vi "laneleftright5.vi"(11 "update":bool=TRUE) -> ()   [LabVIEW 2015]
uses:
  G_SEN.vi
  <vilib>/Analysis/1siggen.llb/Ramp Pattern by Delta.vi
  G_ALL.vi
  <vilib>/Analysis/polynomials.llb/nth Derivative of Polynomial (DBL).vi
  <vilib>/Analysis/polynomials.llb/Scalar Polynomial Evaluation (DBL).vi
  G_LCM.vi
  <vilib>/Analysis/NI_AALPro.lvlib
  <vilib>/Analysis/NI_AALBase.lvlib
panel:
  in  "y limit":dbl=0.01
  in  "d_safe front":dbl=0.5
  out "idxfront":i32=30
  out "h_rf":dbl[](array[numeric])=[-0.9500104358126387, -0.8152801995859489, -0.6832149509832309, -0.5579658214676491, -0.43634713174659895, -0.3636177945739105, -0.4219341557757026, -0.4254071654192556, -0.43418280012028193, -0.4285800458197435, -0.4285800458197435, -0.47492259541262927, -0.43011998989542144, -0.448140819410384, -0.42370272779821094, -0.4351070943600193, -0.3916639450286278, -0.31695052117940714, -0.29608961933059963, -0.29070058934802034, -0.19489158382745403, -0.13694705181123534, -0.0036604327923040465, 0.15093015758716827, 0.24134113354650677, 0.4371774287913892, 0.5886484511821607, 0.5886484511821607, 0.7188655986278671, 0.8431460626855709, 0.9539279580870911, 1.0615621391385646, 1.142586619661877, 1.1293783256575063, 1.1293783256600938, 1.1293783256589616, 1.129378308345949, 1.1293783256583803, 1.1293783256589178, 1.2328992187190753, 1.2383213544784377, 1.2299347078478895, 1.2485889663962422, 1.2492445630317817, 1.2507974714580428, 1.2535353037498, 1.2535353037498, 1.2548915682041502, 1.2388573722116965, 1.2551948137598792, 1.2561989169947274, 1.2545138672661875, 1.2372556012572844, 1.2374470995854208, 1.2497004386998842, 1.258883376955003, 1.238295612670253, 1.249261743063205, 1.2490590423907508, 1.2394351036162379, 1.249147146451496, 1.2523281510667994, 1.2568185177320512, 1.2637485927398984, 1.2729524270473782, 1.2872258426538232, 1.3082533285080937, 1.3356267808199382, 1.3717983894543175, 1.4090203881905266, 1.496939359193244, 1.5483512846148995, 1.5906635102611244, 1.5906635102611244, 1.5906635102611244, 1.5906635102611244, 1.5906635102611244, 1.5906635102611244, 1.5906635102611244, 1.5906635102611244, 1.5906635102611244]
  out "h_lf":dbl[](array[numeric])=[-1.07768170874119, -0.9500104358126387, -0.8152801995859489, -0.6832149509832309, -0.5579658214676491, -0.43634713174659895, -0.3636177945739105, -0.38220962901672345, -0.4254071654192556, -0.43418280012028193, -0.4285800458197435, -0.47492259541262927, -0.43011998989542144, -0.448140819410384, -0.42370272779821094, -0.4351070943600193, -0.3916639450286278, -0.3566256576667743, -0.31695052117940714, -0.29608961933059963, -0.29070058934802034, -0.19489158382745403, -0.13694705181123534, -0.0036604327923040465, 0.15093015758716827, 0.15093015758716827, 0.24134113354650677, 0.4371774287913892, 0.5886484511821607, 0.7188655986278671, 0.8431460626855709, 0.9539279580870911, 1.0615621391385646, 1.142586619661877, 1.1504547666405178, 1.1293783256600938, 1.1293783256589616, 1.1293783256583803, 1.1293783256589178, 1.2328992187190753, 1.2383213544784377, 1.2299347078478895, 1.2299347078478895, 1.2485889663962422, 1.2492445630317817, 1.2507974714580428, 1.2535353037498, 1.2548915682041502, 1.2388573722116965, 1.2551948137598792, 1.2561989169947274, 1.2545138672661875, 1.2372556012572844, 1.2374470995854208, 1.2497004386998842, 1.258883376955003, 1.238295612670253, 1.249261743063205, 1.2490590423907508, 1.2394351036162379, 1.249147146451496, 1.2523281510667994, 1.2568185177320512, 1.2637485927398984, 1.2729524270473782, 1.2872258426538232, 1.3082533285080937, 1.3356267808199382, 1.3717983894543175, 1.4090203881905266, 1.4509264137298254, 1.496939359193244, 1.5483512846148995, 1.5906635102611244, 1.5906635102611244, 1.5906635102611244, 1.5906635102611244, 1.5906635102611244, 1.5906635102611244, 1.5906635102611244, 1.5906635102611244]
  out "size limit":i32=75
  out "sorted array":dbl[](array[numeric])=[3.1256999216175574, 3.1400636936215167, 3.178049716414141, 3.178049716414141, 3.1953090617340916, 3.2015621187164243, 3.2015621187164247, 3.2015621187164247, 3.22490309931942, 3.228002478313795, 3.2280024783137953, 3.2310988842807027, 3.23882694814033, 3.2557641192199416, 3.2557641192199416, 3.2557641192199416, 3.2572994949804666, 3.264965543462902, 3.269556544854363, 3.2756678708318403, 3.2756678708318403, 3.2893768406797053, 3.2893768406797057, 3.298484500494129, 3.298484500494129, 3.298484500494129, 3.301514803843836, 3.306055050963308, 3.3105890714493698, 3.3120990323358392, 3.3136083051561784, 3.3241540277189325, 3.3241540277189325, 3.3241540277189325, 3.3241540277189325, 3.3241540277189325, 3.324154027718933, 3.3376638536557275, 3.3526109228480423, 3.3526109228480423, 3.3526109228480423, 3.3526109228480423, 3.3541019662496847, 3.3541019662496847, 3.361547262794322, 3.361547262794323, 3.383784863137726, 3.3837848631377265, 3.3837848631377265, 3.4, 3.4000000000000004, 3.4000000000000004, 3.400000000000001, 3.4014702703389896, 3.40147027033899, 3.4014702703389905, 3.4132096331752027, 3.417601498127013, 3.417601498127013, 3.417601498127013, 3.4438350715445134, 3.448187929913334, 3.448187929913334, 3.4481879299133342, 3.453983207834109, 3.4669871646719437, 3.4669871646719437, 3.4785054261852175, 3.4785054261852175, 3.4885527085024823, 3.4928498393145966, 3.4985711369071804, 3.511409973215888, 3.5227829907617076, 3.534119409414459, 3.535533905932738, 3.5510561809129415, 3.5777087639996643, 3.580502757993632, 3.5846896657869842, 3.6055512754639896, 3.6235341863986887, 3.635931792539569, 3.6400549446402595, 3.6619666847201118, 3.6878177829171555, 3.7013511046643504, 3.720215047547655, 3.753664875824692, 3.764306044943743, 3.8288379438153295]
  out "element":dbl=2.140625
  out "size(s) 4":i32=91
  out "size(s) 3":i32=52
  in  "x limit":dbl=0.01
  in  "x_gain":dbl=0.5
  out "xr":dbl[](array[numeric])=[2.3000000000000003, 2.3000000000000003, 2.3000000000000003, 2.3000000000000003, 2.3000000000000003, 2.3000000000000003, 2.2, 2.2, 2.2, 2.2, 2.2, 2.2, 2.2, 2.2, 2.2, 2.1, 2.1, 2.1, 2.1, 2.1, 2.1, 2.0, 2.0, 1.9000000000000001, 1.9000000000000001, 1.8, 1.8, 1.8, 1.8, 1.8, 1.7000000000000002, 1.7000000000000002, 1.7000000000000002, 1.7000000000000002, 1.7000000000000002, 1.7000000000000002, 1.7000000000000002, 1.7000000000000002, 1.7000000000000002, 1.7000000000000002, 1.7000000000000002, 1.7000000000000002, 1.7000000000000002, 1.7000000000000002, 1.6, 1.6, 1.6, 1.6, 1.6, 1.6]
  out "yr":dbl[](array[numeric])=[-2.0, -2.1, -2.2, -2.3000000000000003, -2.4000000000000004, -2.5, 1.7000000000000002, 1.6, 1.5, -1.7000000000000002, -1.8, -1.9000000000000001, -2.0, -2.1, -2.2, 1.5, -1.5, -1.6, -1.7000000000000002, -1.8, -1.9000000000000001, -1.5, -1.6, -1.1, -1.2000000000000002, -0.6000000000000001, -0.7000000000000001, -0.8, -1.1, -1.2000000000000002, 0.8, 0.7000000000000001, 0.6000000000000001, 0.5, 0.4, 0.30000000000000004, -0.1, -0.2, -0.30000000000000004, -0.4, -0.5, -0.6000000000000001, -0.7000000000000001, -0.8, 0.4, 0.30000000000000004, 0.2, -0.1, -0.2, -0.30000000000000004]
  out "yl":dbl[](array[numeric])=[-4.800000000000001, -4.9, -5.0, -4.4, -4.5, -4.6000000000000005, -4.7, -4.800000000000001, -4.9, -5.0, -4.1000000000000005, -4.2, -4.3, -4.4, -4.5, -4.6000000000000005, -4.7, -3.7, -3.8000000000000003, -3.9000000000000004, -4.0, -4.1000000000000005, -4.2, -4.3, -4.4, -3.5, -3.6, -3.7, -3.8000000000000003, -3.9000000000000004, -4.0, -4.1000000000000005, -3.0, -3.1, -3.2, -3.3000000000000003, -3.4000000000000004, -3.5, -3.6, -3.7, -2.7, -2.8000000000000003, -2.9000000000000004, -3.0, -3.1, -3.2, -3.3000000000000003, -2.3000000000000003, -2.4000000000000004, -2.5, -2.6, -2.7, -2.8000000000000003, -1.9000000000000001, -2.0, -2.1, -2.2, -2.3000000000000003, -2.4000000000000004, -2.5, -2.6, -1.2000000000000002, -1.3, -1.5, -1.6, -1.7000000000000002, -1.8, -1.9000000000000001, -2.0, -2.1, -2.2, -1.1, -1.2000000000000002, -1.4000000000000001, -1.5, -1.6, -1.7000000000000002, -0.8, -0.9, -1.1, -0.4, -0.5, -0.6000000000000001, -0.7000000000000001, -0.8, -0.9, -0.2, -0.30000000000000004, -0.4]
  out "xl":dbl[](array[numeric])=[-0.5, -0.5, -0.5, -0.6000000000000001, -0.6000000000000001, -0.6000000000000001, -0.6000000000000001, -0.6000000000000001, -0.6000000000000001, -0.6000000000000001, -0.7000000000000001, -0.7000000000000001, -0.7000000000000001, -0.7000000000000001, -0.7000000000000001, -0.7000000000000001, -0.7000000000000001, -0.8, -0.8, -0.8, -0.8, -0.8, -0.8, -0.8, -0.8, -0.9, -0.9, -0.9, -0.9, -0.9, -0.9, -0.9, -1.0, -1.0, -1.0, -1.0, -1.0, -1.0, -1.0, -1.0, -1.1, -1.1, -1.1, -1.1, -1.1, -1.1, -1.1, -1.2000000000000002, -1.2000000000000002, -1.2000000000000002, -1.2000000000000002, -1.2000000000000002, -1.2000000000000002, -1.3, -1.3, -1.3, -1.3, -1.3, -1.3, -1.3, -1.3, -1.4000000000000001, -1.4000000000000001, -1.4000000000000001, -1.4000000000000001, -1.4000000000000001, -1.4000000000000001, -1.4000000000000001, -1.4000000000000001, -1.4000000000000001, -1.4000000000000001, -1.5, -1.5, -1.5, -1.5, -1.5, -1.5, -1.6, -1.6, -1.6, -1.7000000000000002, -1.7000000000000002, -1.7000000000000002, -1.7000000000000002, -1.7000000000000002, -1.7000000000000002, -1.8, -1.8, -1.8]
  out "lf_shift":dbl
  out "lr_shift":dbl
  out "rf_shift":dbl
  out "rr_shift":dbl
  in  "y_gain":dbl=0.5
  out "y_shift":dbl format="%#_13g"
  out "x_shift":dbl format="%#_13g"
  in  "d_safe":dbl=0.25
  out "R0":dbl=3.023957560629749
  out "y_ramp":dbl[](array[numeric])=[-1.0, -0.75, -0.5, -0.25, 0.0, 0.25, 0.5, 0.75, 1.0, 1.25, 1.5, 1.75, 2.0, 2.25, 2.5, 2.75, 3.0, 3.25, 3.5, 3.75, 4.0, 4.25, 4.5, 4.75, 5.0, 5.25, 5.5, 5.75, 6.0]
  out "y_car":dbl[](array[numeric])=[0.0, 3.2, 3.2, 0.0, 0.0]
  out "x_car":dbl[](array[numeric])=[0.8, 0.8, -0.8, -0.8, 0.8]
  out "x_rf":dbl[](array[numeric])=[4.538572328164872, 4.118234620393652, 3.7108458254827896, 3.3870811007829085, 3.120851291928107, 2.916943626318998, 2.7777005691770915, 2.725587769939431, 2.739475625042867, 2.8048150174077966, 2.925745330134693, 2.950997308985372, 2.7112467821790673, 2.394172481092407, 2.174401406783209, 1.9364338560710306, 1.7440716120528545, 1.385310657465475, 1.3006647210601057, 1.0310989075140025, 0.886404618470291, 0.643840438515097, 0.5740896815265153, 0.49712084094748343, 0.45274653237776485, 0.36494746145204304, 0.2359651958610256, 0.40853962746891925, 0.501296155076003, 0.865183184427989, 1.3470915265169374, 1.6921924502018477, 2.350947359675299, 2.926007032436896, 3.472919068553876, 4.01553923764964, 4.540771553603303, 5.060339948090165, 5.558610823136398, 6.019770740590945, 6.466417913813986, 6.886028933795981, 7.305639953774969, 7.725250962609034, 8.144861995684934, 8.564473015664918, 9.033292240733939, 9.507748305528745, 9.982559003445736, 10.465812099477526, 10.944605083330368, 11.422232043345485, 11.918421793799222, 12.414200190202452, 12.899637481676528, 13.37678754684273, 13.874783465668319, 14.370744561954087, 14.868407110563963, 15.347734850377055, 15.829260577613933, 16.33800747711995, 16.840800167460728, 17.330629454236842, 17.83149600020578, 18.307170795470793, 18.793936003289474, 19.282694540287146, 19.78369621145204, 20.267635515491328, 20.756809613631752, 21.25179974157784, 21.74713849772317, 22.236508427679524, 22.722656802659756, 23.209593805045373, 23.694584083823898, 24.18159320732069, 24.656670896067542, 25.139986749461006, 25.646977091436657]
  out "y_rf":dbl[](array[numeric])=[-11.133801995366914, -10.775342355485478, -10.460977313011862, -10.008167510844103, -9.519733334433447, -9.006779742303703, -8.476797423718132, -7.920018039425989, -7.363784000331509, -6.820753362891501, -6.29243806249853, -5.801400680342903, -5.33902916891923, -4.892670984988988, -4.430237539433438, -3.9731282342132452, -3.5156906037336335, -3.0892706515763058, -2.6129748065047353, -2.163986278307514, -1.6831045571753158, -1.2341811741681994, -0.7562032880817622, -0.27746062806621064, 0.20341311916780747, 0.6846965145469994, 1.1665722299824774, 1.6449603307709209, 2.125056894695668, 2.5475589084455996, 2.8962835690170365, 3.265562716322244, 3.4006089292605273, 3.512279221773241, 3.5953374904708157, 3.622437769324544, 3.623063809872327, 3.5757747817018526, 3.56036016701454, 3.743209849888086, 4.016917878895559, 4.215189945468877, 4.413462012052612, 4.61173413464184, 4.810006155024352, 5.008278221603526, 4.868806594115014, 5.017139252390996, 5.209509379461617, 5.317736171223016, 5.47536534066575, 5.629232093137066, 5.784437062614739, 5.942659837296325, 6.155411787532055, 6.264698912841051, 6.42392237988264, 6.590981837822474, 6.812082411109792, 6.977514156959353, 7.102822406709091, 7.24110252096422, 7.472616124159055, 7.604691291930131, 7.772210321235591, 7.963262450759516, 8.097906275068672, 8.250045548981548, 8.40009947677207, 8.53394808955574, 8.658191795172698, 8.762449905848245, 8.8369058516278, 8.878040735642243, 8.876062057147013, 8.853346181102042, 8.797375639621363, 8.708634139574771, 8.579950576586779, 8.456123819728742, 8.446050024161806]
  out "y_rr":dbl[](array[numeric])=[-10.70948639810373, -10.768851501394227, -10.773698390308322, -10.742191022481514, -10.657439960127398, -10.52156928101113, -10.338156146215423, -10.114144305421542, -9.845534928412233, -9.535421794598271, -9.192602940142088, -8.792172667355606, -8.308126041009189, -7.812026379085751, -7.345024018399936, -6.876213405347107, -6.426272269508127, -5.935120632545394, -5.521505119616947, -5.047999798768626, -4.600137704349835, -4.136020874717464, -3.7138838228732727, -3.2761172269068966, -2.837195735363109, -2.3760547770738345, -1.8991663469164366, -1.4944594171009975, -1.0449827814742285, -0.6524196535491742, -0.2673377084370725, 0.15830412292045987, 0.5015679626686349, 0.8508652409058738, 1.187167083685631, 1.4940639050112943, 1.771916455237049, 2.0157467968022704, 2.231583141944811, 2.437378476871852, 2.6498075579368594, 2.848079624517664, 3.0463516910981228, 3.2446237635961372, 3.442895834068181, 3.6411679006489104, 3.8079942899104933, 3.972712173496366, 4.139751736152054, 4.304420660079245, 4.464039995334728, 4.6226225761415085, 4.786147622632705, 4.948494763708864, 5.1126061835115255, 5.271456251848721, 5.43373465243814, 5.595668001049872, 5.764432278430686, 5.930443066452188, 6.09288119931919, 6.259087021699353, 6.428111182822922, 6.59341810511168, 6.760321754935594, 6.922204842602915, 7.086285179001638, 7.248086732121628, 7.411797351666064, 7.566761628321898, 7.719120690821865, 7.867136904452785, 8.006386664257533, 8.132415557859344, 8.243463199248932, 8.337918310717816, 8.414709864120713, 8.472506653347954, 8.508132472051695, 8.519694624675884, 8.509620829108949]
  out "x_rr":dbl[](array[numeric])=[7.710315740535928, 7.318228037388939, 6.895528781102477, 6.501757566222534, 6.111774833888363, 5.735704462825447, 5.380649609435707, 5.054924570161421, 4.7596024356590885, 4.499092239675365, 4.278166744665951, 4.089102278529083, 3.904755795193055, 3.7046548666886947, 3.495014818056198, 3.282575189342792, 3.0739266292849514, 2.848573410978404, 2.6350002926864415, 2.4176291141079678, 2.2020480421551136, 1.9926645012883535, 1.7956157164989206, 1.6142862728460952, 1.4500919057305408, 1.2986505892402076, 1.1531603649029383, 1.028252179118328, 0.9381582059669654, 0.8768965432058912, 0.8659466285499812, 0.9273761103327463, 0.9961184132684305, 1.1492471661511572, 1.365618593566012, 1.6259734415878775, 1.9305505914189107, 2.2663620157631854, 2.647536860206764, 3.0983319811358476, 3.573148246062948, 3.9927592660414053, 4.412370286021941, 4.8319813185248055, 5.251592327932702, 5.67120334791195, 6.014239863704302, 6.482988467645475, 6.9666646776145456, 7.430488117614067, 7.908617427576298, 8.384677553250869, 8.878122763437181, 9.372550012016466, 9.874318246914124, 10.334836032372968, 10.831836166680331, 11.329470097797818, 11.84476209179978, 12.323889263806183, 12.792812198731816, 13.29241302624446, 13.816067216021146, 14.294624424329601, 14.795696018423165, 15.281249604081424, 15.758046881797691, 16.24360281259667, 16.740135975558726, 17.21729941118971, 17.697701008012572, 18.179599450331803, 18.656792581905684, 19.124588908434816, 19.585808275078925, 20.051376885574644, 20.517546642391945, 20.99031700331575, 21.45747691009842, 21.940618256655217, 22.447608598630868]
  out "x_lr":dbl[](array[numeric])=[7.9224735391675205, 7.321473464434564, 6.739168242454245, 6.134745810403829, 5.542921521041388, 4.978309693471735, 4.449970248187061, 3.9578614371636447, 3.5187269716187273, 3.14175802382198, 2.8280843058441714, 2.5937162850227318, 2.4202073591480753, 2.244977169640313, 2.0376215785729492, 1.8310326037758613, 1.6186357963977047, 1.42564842049386, 1.1807351361303358, 0.9756223538774118, 0.7435314685678545, 0.5417446510137208, 0.31677544910316535, 0.1149579734257522, -0.0702125215349173, -0.23172505657020925, -0.37970892354651875, -0.5414576948176312, -0.6468616321179829, -0.7230927377914959, -0.7158640101770734, -0.6262531863681458, -0.45340207002751576, -0.18145982428252616, 0.16153339017341928, 0.5617865094312524, 1.0049769141012719, 1.4863480233133943, 1.9831483476718994, 2.4454162946277305, 2.889593085583598, 3.309204105565798, 3.7288151255446973, 4.148426133001953, 4.568037167454616, 4.987648187434642, 5.483833711602041, 5.960774928198159, 6.431785855959763, 6.923830362042183, 7.402954754910787, 7.88137279475309, 8.378978043446166, 8.875467475222736, 9.352915444903859, 9.838214701876803, 10.336742302958081, 10.831813179411517, 11.320937025460228, 11.8003537185526, 12.287841595036866, 12.801405276612027, 13.293814745353078, 13.788987830920377, 14.289751735273168, 14.760720800003124, 15.252236333764175, 15.74262340416671, 16.245984913005724, 16.733706180572792, 17.228165455837157, 17.73194294963407, 18.24153298822055, 18.751776319543367, 19.26950884612988, 19.79366295038253, 20.326213754641618, 20.87225326020234, 21.42156785783088, 21.97240365912879, 22.479394001104442]
  out "y_lr":dbl[](array[numeric])=[-12.295358104289258, -12.368848209891869, -12.366039868118165, -12.299529255201328, -12.152901731107526, -11.930949699264355, -11.63963066634473, -11.278812705532536, -10.855598333720343, -10.382560405732054, -9.868813647407716, -9.361225152127462, -8.904880547516182, -8.467267571883895, -8.005330724036432, -7.549284071982989, -7.0911997781241745, -6.666752009301859, -6.188672905430115, -5.741264902065608, -5.257959416192246, -4.810432906104093, -4.324646840359476, -3.834699942856202, -3.3358684220394967, -2.8429063409679163, -2.357763931437393, -1.8043156929257018, -1.2634138069197096, -0.6582763329381254, -0.026765259453594398, 0.5407122928550108, 1.178982435872069, 1.7392451740487433, 2.240817321179563, 2.6888468030421757, 3.0770269363292453, 3.4127357629657604, 3.6871201234096276, 3.898097856599401, 4.096442391812379, 4.294714458394951, 4.492986524974636, 4.691258585638252, 4.889530667944297, 5.087802734525394, 5.317520478425312, 5.485092092438001, 5.64769889906765, 5.822082651010975, 5.982033823211763, 6.141399821188817, 6.306297137813725, 6.469319852801857, 6.625265800892727, 6.792432009083602, 6.955208301932135, 7.116305233128007, 7.276254787812777, 7.442365859737624, 7.611105388760248, 7.781884247137096, 7.940477658542712, 8.1114206200653, 8.278221745826903, 8.4351654382976, 8.604229739747527, 8.767632595966866, 8.93357746961272, 9.091929680472706, 9.248674993631454, 9.403237050075806, 9.551559622166277, 9.688375317481698, 9.811887463039348, 9.917026770453182, 10.003228584836691, 10.068144755350426, 10.107729465036254, 10.119378871078778, 10.109305075511843]
  out "af":dbl=3.2
  out "y_lf":dbl[](array[numeric])=[-12.719673701552441, -12.375339063983121, -12.053318790821704, -11.565505743563916, -11.015195105413575, -10.416160160556927, -9.77827194384744, -9.084686439536984, -8.37384740563962, -7.667891974025285, -6.968648769764158, -6.370453165114759, -5.935783675426223, -5.547912177787132, -5.090544245069932, -4.646198900849126, -4.180618112349682, -3.82090202833277, -3.280142592317903, -2.8572513816044967, -2.340926269017727, -1.9085932055548271, -1.3669663055679653, -0.8360433440155162, -0.2952595675085803, 0.21784495065291676, 0.7079746454615212, 1.3351040549462165, 1.906625869250187, 2.5417022290566487, 3.1368560180005147, 3.6479708862567946, 4.078023402463962, 4.40065915491611, 4.648987727964748, 4.817220667355426, 4.928174290964523, 4.9727637478653435, 5.0158971484793575, 5.2039292296156345, 5.463552712771079, 5.661824779346166, 5.860096845929126, 6.058368956683955, 6.256640988900468, 6.45491305548001, 6.378332782629832, 6.529519171332631, 6.717456542377213, 6.835398162154745, 6.993359168542785, 7.148009338184375, 7.304586577795758, 7.4634849263893175, 7.668071404913257, 7.785674670075932, 7.945396029376635, 8.111619069900609, 8.323904920491882, 8.489436950244789, 8.62104659615015, 8.763899746401965, 8.984982599878846, 9.122693806883749, 9.290110312126899, 9.476223046454201, 9.615850835814562, 9.769591412826784, 9.921879594718726, 10.059116141706546, 10.187746097982288, 10.298550051471265, 10.382078809536544, 10.434000495264597, 10.44448632093743, 10.432454640837406, 10.385894360337339, 10.304272241577243, 10.179547569571339, 10.055808066131636, 10.0457342705647]
  out "x_lf":dbl[](array[numeric])=[4.750730126796465, 4.121480047439278, 3.5544852868345593, 3.0200693449642024, 2.5519979790811314, 2.159548856965284, 1.847021207928445, 1.628524636941655, 1.4986001610025053, 1.4474808015544118, 1.4756628913129135, 1.455611315479021, 1.226698346134088, 0.9344947840440256, 0.7170081672999595, 0.48489127050409975, 0.28878077916560807, -0.037614333019069246, -0.15360043549600033, -0.4109078527165533, -0.5721119551169682, -0.8070794117595357, -0.90475058586924, -1.0022074584728595, -1.0675578948876934, -1.1654281843583738, -1.2969040925884314, -1.16117024646704, -1.0837236830089454, -0.734806096569398, -0.23471911221011726, 0.13856315350095594, 0.9014268763793528, 1.5953000420032126, 2.2688338651612834, 2.951352305493015, 3.615197876285664, 4.280325955640375, 4.894222310601533, 5.366855054082828, 5.782862753334636, 6.202473773320374, 6.6220847932977245, 7.041695777086183, 7.461306835206849, 7.88091785518761, 8.502886088631676, 8.98553476608143, 9.447680181790954, 9.95915434390564, 10.438942410664858, 10.918927284847708, 11.419277073808205, 11.917117653408722, 12.378234679666264, 12.880166216346565, 13.379689601946069, 13.873087643567787, 14.34458204422441, 14.824199305123472, 15.324289973918983, 15.846999727487516, 16.31854769679266, 16.824992860827617, 17.325551717055784, 17.786641991392493, 18.288125455255955, 18.781715131857183, 19.289545148899034, 19.784042284874406, 20.287274061456333, 20.804143240880112, 21.33187890403804, 21.863695838788075, 22.406357373710716, 22.951879869853258, 23.50325119607357, 24.063529464207285, 24.6207618438, 25.171772151934576, 25.678762493910227]
  out "h_path":dbl[](array[numeric])=[-1.7037866247771944, -1.5728247200893424, -1.4729147677282362, -1.3393532640375114, -1.2073117198254844, -1.07768170874119, -0.9500104358126387, -0.8152801995859489, -0.6832149509832309, -0.5579658214676491, -0.43634713174659895, -0.3636177945739105, -0.38220962901672345, -0.4219341557757026, -0.4254071654192556, -0.43418280012028193, -0.4285800458197435, -0.47492259541262927, -0.43011998989542144, -0.448140819410384, -0.42370272779821094, -0.4351070943600193, -0.3916639450286278, -0.3566256576667743, -0.31695052117940714, -0.29608961933059963, -0.29070058934802034, -0.19489158382745403, -0.13694705181123534, -0.0036604327923040465, 0.15093015758716827, 0.24134113354650677, 0.4371774287913892, 0.5886484511821607, 0.7188655986278671, 0.8431460626855709, 0.9539279580870911, 1.0615621391385646, 1.142586619661877, 1.1504547666405178, 1.1293783256575063, 1.1293783256600938, 1.1293783256589616, 1.129378308345949, 1.1293783256583803, 1.1293783256589178, 1.2328992187190753, 1.2383213544784377, 1.2299347078478895, 1.2485889663962422, 1.2492445630317817, 1.2507974714580428, 1.2535353037498, 1.2548915682041502, 1.2388573722116965, 1.2551948137598792, 1.2561989169947274, 1.2545138672661875, 1.2372556012572844, 1.2374470995854208, 1.2497004386998842, 1.258883376955003, 1.238295612670253, 1.249261743063205, 1.2490590423907508, 1.2394351036162379, 1.249147146451496, 1.2523281510667994, 1.2568185177320512, 1.2637485927398984, 1.2729524270473782, 1.2872258426538232, 1.3082533285080937, 1.3356267808199382, 1.3717983894543175, 1.4090203881905266, 1.4509264137298254, 1.496939359193244, 1.5483512846148995, 1.5906635102611244, 1.5906635102611244]
  out "x_path":dbl[](array[numeric])=[7.816394639851724, 7.319850750911751, 6.817348511778361, 6.318251688313182, 5.827348177464875, 5.357007078148591, 4.915309928811384, 4.506393003662533, 4.139164703638908, 3.8204251317486726, 3.553125525255061, 3.3414092817759076, 3.162481577170565, 2.974816018164504, 2.7663181983145737, 2.5568038965593267, 2.346281212841328, 2.137110915736132, 1.9078677144083886, 1.6966257339926898, 1.4727897553614842, 1.267204576151037, 1.056195582801043, 0.8646221231359237, 0.6899396920978118, 0.5334627663349991, 0.38672572067820976, 0.24339724215034841, 0.1456482869244913, 0.07690190270719764, 0.07504130918645387, 0.15056146198230025, 0.2713581716204574, 0.48389367093431557, 0.7635759918697156, 1.093879975509565, 1.4677637527600913, 1.8763550195382899, 2.3153426039393317, 2.771874137881789, 3.231370665823273, 3.6509816858036017, 4.070592705783319, 4.490203725763379, 4.909814747693659, 5.329425767673296, 5.749036787653171, 6.221881697921817, 6.699225266787154, 7.177159239828125, 7.6557860912435425, 8.133025174001979, 8.628550403441674, 9.124008743619601, 9.613616845908991, 10.086525367124885, 10.584289234819206, 11.080641638604668, 11.582849558630004, 12.062121491179392, 12.540326896884341, 13.046909151428244, 13.554940980687112, 14.041806127624989, 14.542723876848166, 15.020985202042274, 15.505141607780933, 15.99311310838169, 16.493060444282225, 16.97550279588125, 17.462933231924865, 17.955771199982937, 18.449162785063116, 18.938182613989092, 19.427658560604403, 19.922519917978587, 20.42188019851678, 20.931285131759044, 21.43952238396465, 21.956510957892004, 22.463501299867655]
  out "y_path":dbl[](array[numeric])=[-11.502422251196494, -11.568849855643048, -11.569869129213243, -11.520860138841421, -11.405170845617462, -11.226259490137743, -10.988893406280077, -10.696478505477039, -10.350566631066288, -9.958991100165163, -9.530708293774902, -9.076698909741534, -8.606503294262685, -8.139646975484823, -7.675177371218184, -7.212748738665048, -6.758736023816151, -6.300936320923626, -5.855089012523531, -5.394632350417117, -4.92904856027104, -4.473226890410778, -4.019265331616374, -3.5554085848815493, -3.086532078701303, -2.6094805590208754, -2.1284651391769147, -1.6493875550133497, -1.154198294196969, -0.6553479932436498, -0.14705148394533343, 0.3495082078877353, 0.840275199270352, 1.2950552074773085, 1.7139922024325969, 2.091455354026735, 2.424471695783147, 2.7142412798840154, 2.9593516326772193, 3.1677381667356266, 3.373124974874619, 3.571397041456308, 3.76966910803638, 3.9679411746171946, 4.166213251006239, 4.364485317587152, 4.562757384167902, 4.728902132967184, 4.893725317609852, 5.06325165554511, 5.223036909273246, 5.382011198665163, 5.546222380223215, 5.708907308255361, 5.868935992202126, 6.031944130466162, 6.194471477185138, 6.35598661708894, 6.520343533121731, 6.686404463094906, 6.851993294039719, 7.0204856344182245, 7.184294420682817, 7.35241936258849, 7.5192717503812485, 7.678685140450257, 7.845257459374583, 8.007859664044247, 8.172687410639393, 8.329345654397303, 8.483897842226659, 8.635186977264295, 8.778973143211905, 8.910395437670521, 9.02767533114414, 9.127472540585499, 9.208969224478702, 9.27032570434919, 9.307930968543975, 9.319536747877331, 9.309462952310396]
  out "gap":dbl=0.8
  out "theta":dbl[](array[numeric])=[-3.141592653589793, -3.1315926535897933, -3.121592653589793, -3.1115926535897933, -3.101592653589793, -3.0915926535897933, -3.081592653589793, -3.0715926535897933, -3.061592653589793, -3.0515926535897933, -3.041592653589793, -3.0315926535897932, -3.021592653589793, -3.0115926535897932, -3.001592653589793, -2.991592653589793, -2.981592653589793, -2.971592653589793, -2.961592653589793, -2.951592653589793, -2.941592653589793, -2.931592653589793, -2.921592653589793, -2.911592653589793, -2.901592653589793, -2.891592653589793, -2.8815926535897933, -2.871592653589793, -2.861592653589793, -2.851592653589793, -2.8415926535897933, -2.831592653589793, -2.8215926535897933, -2.811592653589793, -2.8015926535897933, -2.791592653589793, -2.7815926535897932, -2.771592653589793, -2.7615926535897932, -2.751592653589793, -2.741592653589793, -2.731592653589793, -2.721592653589793, -2.711592653589793, -2.701592653589793, -2.691592653589793, -2.681592653589793, -2.671592653589793, -2.661592653589793, -2.651592653589793, -2.641592653589793, -2.6315926535897933, -2.621592653589793, -2.611592653589793, -2.601592653589793, -2.5915926535897933, -2.581592653589793, -2.571592653589793, -2.561592653589793, -2.5515926535897933, -2.541592653589793, -2.5315926535897932, -2.521592653589793, -2.5115926535897932, -2.501592653589793, -2.491592653589793, -2.481592653589793, -2.471592653589793, -2.461592653589793, -2.451592653589793, -2.441592653589793, -2.431592653589793, -2.4215926535897934, -2.411592653589793, -2.401592653589793, -2.391592653589793, -2.3815926535897933, -2.371592653589793, -2.361592653589793, -2.351592653589793, -2.3415926535897933, -2.331592653589793, -2.321592653589793, -2.311592653589793, -2.3015926535897933, -2.291592653589793, -2.2815926535897932, -2.271592653589793, -2.2615926535897932, -2.251592653589793, -2.241592653589793, -2.231592653589793, -2.221592653589793, -2.211592653589793, -2.201592653589793, -2.191592653589793, -2.181592653589793, -2.1715926535897934, -2.161592653589793, -2.151592653589793, -2.141592653589793, -2.1315926535897933, -2.121592653589793, -2.111592653589793, -2.101592653589793, -2.0915926535897933, -2.081592653589793, -2.071592653589793, -2.061592653589793, -2.0515926535897933, -2.041592653589793, -2.031592653589793, -2.021592653589793, -2.0115926535897932, -2.001592653589793, -1.991592653589793, -1.9815926535897932, -1.9715926535897932, -1.9615926535897932, -1.9515926535897932, -1.9415926535897932, -1.9315926535897932, -1.9215926535897931, -1.9115926535897931, -1.9015926535897931, -1.8915926535897931, -1.881592653589793, -1.871592653589793, -1.861592653589793, -1.851592653589793, -1.841592653589793, -1.831592653589793, -1.821592653589793, -1.811592653589793, -1.801592653589793, -1.791592653589793, -1.781592653589793, -1.771592653589793, -1.761592653589793, -1.751592653589793, -1.741592653589793, -1.7315926535897932, -1.7215926535897932, -1.7115926535897932, -1.7015926535897932, -1.6915926535897932, -1.6815926535897932, -1.6715926535897931, -1.6615926535897931, -1.6515926535897931, -1.6415926535897931, -1.631592653589793, -1.621592653589793, -1.611592653589793, -1.601592653589793, -1.591592653589793, -1.581592653589793, -1.571592653589793, -1.561592653589793, -1.551592653589793, -1.541592653589793, -1.531592653589793, -1.521592653589793, -1.511592653589793, -1.501592653589793, -1.491592653589793, -1.481592653589793, -1.4715926535897932, -1.4615926535897932, -1.4515926535897932, -1.4415926535897932, -1.4315926535897932, -1.4215926535897931, -1.4115926535897931, -1.4015926535897931, -1.3915926535897931, -1.381592653589793, -1.371592653589793, -1.361592653589793, -1.351592653589793, -1.341592653589793, -1.331592653589793, -1.321592653589793, -1.311592653589793, -1.301592653589793, -1.291592653589793, -1.281592653589793, -1.271592653589793, -1.261592653589793, -1.251592653589793, -1.241592653589793, -1.231592653589793, -1.2215926535897932, -1.2115926535897932, -1.2015926535897932, -1.1915926535897932, -1.1815926535897932, -1.1715926535897931, -1.1615926535897931, -1.1515926535897931, -1.1415926535897931, -1.1315926535897929, -1.121592653589793, -1.1115926535897929, -1.101592653589793, -1.0915926535897933, -1.081592653589793, -1.0715926535897933, -1.061592653589793, -1.0515926535897933, -1.041592653589793, -1.0315926535897932, -1.021592653589793, -1.0115926535897932, -1.001592653589793, -0.9915926535897932, -0.981592653589793, -0.9715926535897932, -0.961592653589793, -0.9515926535897932, -0.9415926535897929, -0.9315926535897932, -0.9215926535897929, -0.9115926535897931, -0.9015926535897929, -0.8915926535897931, -0.8815926535897929, -0.8715926535897931, -0.8615926535897929, -0.8515926535897931, -0.8415926535897928, -0.8315926535897931, -0.8215926535897933, -0.811592653589793, -0.8015926535897933, -0.791592653589793, -0.7815926535897932, -0.771592653589793, -0.7615926535897932, -0.751592653589793, -0.7415926535897932, -0.731592653589793, -0.7215926535897932, -0.711592653589793, -0.7015926535897932, -0.6915926535897929, -0.6815926535897932, -0.6715926535897929, -0.6615926535897931, -0.6515926535897929, -0.6415926535897931, -0.6315926535897929, -0.6215926535897931, -0.6115926535897929, -0.6015926535897931, -0.5915926535897928, -0.5815926535897931, -0.5715926535897933, -0.561592653589793, -0.5515926535897933, -0.541592653589793, -0.5315926535897932, -0.521592653589793, -0.5115926535897932, -0.501592653589793, -0.4915926535897932, -0.481592653589793, -0.4715926535897932, -0.46159265358979296, -0.45159265358979317, -0.44159265358979294, -0.43159265358979315, -0.4215926535897929, -0.41159265358979313, -0.4015926535897929, -0.3915926535897931, -0.3815926535897929, -0.3715926535897931, -0.36159265358979287, -0.3515926535897931, -0.34159265358979285, -0.33159265358979306, -0.3215926535897933, -0.31159265358979304, -0.30159265358979326, -0.291592653589793, -0.28159265358979324, -0.271592653589793, -0.2615926535897932, -0.251592653589793, -0.2415926535897932, -0.23159265358979297, -0.2215926535897932, -0.21159265358979296, -0.20159265358979317, -0.19159265358979294, -0.18159265358979315, -0.17159265358979292, -0.16159265358979313, -0.1515926535897929, -0.14159265358979312, -0.13159265358979289, -0.1215926535897931, -0.11159265358979287, -0.10159265358979308, -0.09159265358979285, -0.08159265358979306, -0.07159265358979283, -0.061592653589793045, -0.05159265358979326, -0.04159265358979303, -0.03159265358979324, -0.02159265358979301, -0.011592653589793223, -0.0015926535897929917, 0.008407346410206795, 0.018407346410207026, 0.028407346410206813, 0.038407346410207044, 0.04840734641020683, 0.05840734641020706, 0.06840734641020685, 0.07840734641020708, 0.08840734641020687, 0.0984073464102071, 0.10840734641020688, 0.11840734641020711, 0.1284073464102069, 0.13840734641020713, 0.14840734641020692, 0.15840734641020715, 0.16840734641020694, 0.17840734641020717, 0.18840734641020696, 0.19840734641020674, 0.20840734641020697, 0.21840734641020676, 0.228407346410207, 0.23840734641020678, 0.248407346410207, 0.2584073464102068, 0.268407346410207, 0.2784073464102068, 0.28840734641020704, 0.29840734641020683, 0.30840734641020706, 0.31840734641020685, 0.3284073464102071, 0.33840734641020687, 0.3484073464102071, 0.3584073464102069, 0.3684073464102071, 0.3784073464102069, 0.38840734641020713, 0.3984073464102069, 0.40840734641020715, 0.41840734641020694, 0.42840734641020717, 0.43840734641020696, 0.44840734641020674, 0.458407346410207, 0.46840734641020676, 0.478407346410207, 0.4884073464102068, 0.498407346410207, 0.5084073464102068, 0.518407346410207, 0.5284073464102068, 0.538407346410207, 0.5484073464102068, 0.5584073464102071, 0.5684073464102068, 0.5784073464102071, 0.5884073464102069, 0.5984073464102071, 0.6084073464102069, 0.6184073464102071, 0.6284073464102069, 0.6384073464102071, 0.6484073464102069, 0.6584073464102072, 0.6684073464102069, 0.6784073464102072, 0.688407346410207, 0.6984073464102067, 0.708407346410207, 0.7184073464102068, 0.728407346410207, 0.7384073464102068, 0.748407346410207, 0.7584073464102068, 0.768407346410207, 0.7784073464102068, 0.788407346410207, 0.7984073464102068, 0.8084073464102071, 0.8184073464102068, 0.8284073464102071, 0.8384073464102069, 0.8484073464102071, 0.8584073464102069, 0.8684073464102067, 0.8784073464102073, 0.8884073464102071, 0.8984073464102069, 0.9084073464102067, 0.9184073464102074, 0.9284073464102072, 0.938407346410207, 0.9484073464102067, 0.9584073464102065, 0.9684073464102072, 0.978407346410207, 0.9884073464102068, 0.9984073464102066, 1.0084073464102072, 1.018407346410207, 1.0284073464102068, 1.0384073464102066, 1.0484073464102073, 1.058407346410207, 1.0684073464102068, 1.0784073464102066, 1.0884073464102073, 1.098407346410207, 1.1084073464102069, 1.1184073464102067, 1.1284073464102073, 1.1384073464102071, 1.148407346410207, 1.1584073464102067, 1.1684073464102074, 1.1784073464102072, 1.188407346410207, 1.1984073464102067, 1.2084073464102074, 1.2184073464102072, 1.228407346410207, 1.2384073464102068, 1.2484073464102066, 1.2584073464102072, 1.268407346410207, 1.2784073464102068, 1.2884073464102066, 1.2984073464102073, 1.308407346410207, 1.3184073464102068, 1.3284073464102066, 1.3384073464102073, 1.348407346410207, 1.3584073464102069, 1.3684073464102067, 1.3784073464102073, 1.3884073464102071, 1.398407346410207, 1.4084073464102067, 1.4184073464102074, 1.4284073464102072, 1.438407346410207, 1.4484073464102067, 1.4584073464102074, 1.4684073464102072, 1.478407346410207, 1.4884073464102068, 1.4984073464102066, 1.5084073464102072, 1.518407346410207, 1.5284073464102068, 1.5384073464102066, 1.5484073464102073, 1.558407346410207, 1.5684073464102068, 1.5784073464102066, 1.5884073464102073, 1.598407346410207, 1.6084073464102069, 1.6184073464102067, 1.6284073464102073, 1.6384073464102071, 1.648407346410207, 1.6584073464102067, 1.6684073464102074, 1.6784073464102072, 1.688407346410207, 1.6984073464102067, 1.7084073464102074, 1.7184073464102072, 1.728407346410207, 1.7384073464102068, 1.7484073464102066, 1.7584073464102072, 1.768407346410207, 1.7784073464102068, 1.7884073464102066, 1.7984073464102073, 1.808407346410207, 1.8184073464102068, 1.8284073464102066, 1.8384073464102073, 1.848407346410207, 1.8584073464102069, 1.8684073464102067, 1.8784073464102073, 1.8884073464102071, 1.898407346410207, 1.9084073464102067, 1.9184073464102074, 1.9284073464102072, 1.938407346410207, 1.9484073464102067, 1.9584073464102074, 1.9684073464102072, 1.978407346410207, 1.9884073464102068, 1.9984073464102066, 2.0084073464102072, 2.018407346410207, 2.028407346410207, 2.0384073464102066, 2.0484073464102073, 2.058407346410207, 2.068407346410207, 2.0784073464102066, 2.0884073464102073, 2.098407346410207, 2.108407346410207, 2.1184073464102067, 2.1284073464102073, 2.138407346410207, 2.148407346410207, 2.1584073464102067, 2.1684073464102074, 2.178407346410207, 2.188407346410207, 2.1984073464102067, 2.2084073464102074, 2.218407346410207, 2.228407346410207, 2.2384073464102068, 2.2484073464102066, 2.2584073464102072, 2.268407346410207, 2.278407346410207, 2.2884073464102066, 2.2984073464102073, 2.308407346410207, 2.318407346410207, 2.3284073464102066, 2.3384073464102073, 2.348407346410207, 2.358407346410207, 2.3684073464102067, 2.3784073464102073, 2.388407346410207, 2.398407346410207, 2.4084073464102067, 2.4184073464102074, 2.428407346410207, 2.438407346410207, 2.4484073464102067, 2.4584073464102074, 2.468407346410207, 2.478407346410207, 2.4884073464102068, 2.4984073464102066, 2.5084073464102072, 2.518407346410207, 2.528407346410207, 2.5384073464102066, 2.5484073464102073, 2.558407346410207, 2.568407346410207, 2.5784073464102066, 2.5884073464102073, 2.598407346410207, 2.608407346410207, 2.6184073464102067, 2.6284073464102073, 2.638407346410207, 2.648407346410207, 2.6584073464102067, 2.6684073464102074, 2.678407346410207, 2.688407346410207, 2.6984073464102067, 2.7084073464102074, 2.718407346410207, 2.728407346410207, 2.7384073464102068, 2.7484073464102066, 2.7584073464102072, 2.768407346410207, 2.778407346410207, 2.7884073464102066, 2.7984073464102073, 2.808407346410207, 2.818407346410207, 2.8284073464102066, 2.8384073464102073, 2.848407346410207, 2.858407346410207, 2.8684073464102067, 2.8784073464102073, 2.888407346410207, 2.898407346410207, 2.9084073464102067, 2.9184073464102074, 2.928407346410207, 2.938407346410207, 2.9484073464102067, 2.9584073464102074, 2.968407346410207, 2.978407346410207, 2.9884073464102068, 2.9984073464102075, 3.0084073464102072, 3.018407346410207, 3.028407346410207, 3.0384073464102066, 3.0484073464102073, 3.058407346410207, 3.068407346410207, 3.0784073464102066, 3.0884073464102073, 3.098407346410207, 3.108407346410207, 3.1184073464102067, 3.1284073464102073, 3.138407346410207, -3.141592653589793]
  out "y":dbl[](array[numeric])=[3.98, 3.92, 3.9, 3.88, 3.96, 3.94, 3.9, 3.88, 3.98, 3.96, 3.94, 3.88, 3.98, 3.96, 3.94, 3.92, 3.9, 3.98, 3.98, 3.96, 3.94, 4.0200000000000005, 4.0, 3.98, 3.94, 4.0200000000000005, 4.0, 3.98, 3.94, 3.96, 3.94, 4.0200000000000005, 3.96, 4.0600000000000005, 4.04, 4.0, 3.98, 4.0600000000000005, 4.0, 3.98, 4.0600000000000005, 4.04, 4.0200000000000005, -0.24, -0.26, -0.3, -0.32, -0.34, 4.04, 4.0200000000000005, -0.24, -0.26, -0.3, -0.32, -0.34, -0.36, -0.38, -0.24, -0.3, -0.32, -0.34, -0.36, -0.38, -0.4, -0.42, -0.32, -0.36, -0.4, -0.38, -0.42, -0.44, -0.46, -0.48, -0.5, -0.52, -0.54, -0.56, -0.58, -0.6, -0.64, -0.66, -0.68, -0.7000000000000001, -0.4, -0.46, -0.48, -0.52, -0.54, -0.56, -0.6, -0.64, -0.66, -0.7000000000000001, -0.4, -0.42, -0.44, -0.5, -0.54, -0.6, -0.62, -0.64, -0.66, -0.7000000000000001, -0.72, -0.74, -0.76, -0.78, -0.8, -0.8200000000000001, -0.84, -0.68, -0.72, -0.74, -0.76, -0.8, -0.84, 4.1, 4.0600000000000005, 4.04, -0.68, -0.7000000000000001, -0.72, -0.76, -0.8, -0.8200000000000001, -0.84, -0.86, 4.1, 4.08, 4.0600000000000005, 4.04, -0.84, -0.86, 4.1, 4.08, 4.0600000000000005, 4.04, -0.8200000000000001, -0.84, -0.86, 4.1, 4.0600000000000005, 4.04, 4.08, 4.0600000000000005, 4.04, -1.08, -1.1, -1.12, -1.08, -1.1, -1.12, -1.08, -1.1, -1.12, -1.4000000000000001, -1.44, -1.46, -1.48, -1.5, -1.52, -1.08, -1.1, -1.4000000000000001, -1.42, -1.44, -1.5, -1.22, -1.24, -1.4000000000000001, -1.42, -1.44, -1.46, -1.48, -1.52, -1.54, -1.56, -1.6, -1.6600000000000001, -1.68, 4.1, 4.08, -1.24, -1.4000000000000001, -1.42, -1.44, -1.46, -1.5, -1.54, -1.56, -1.6, -1.6400000000000001, -1.6600000000000001, -1.68, -1.7, -1.72, 4.14, 4.1, -1.22, -1.24, -1.54, -1.56, -1.58, -1.62, -1.6400000000000001, -1.68, -1.72, -1.74, -1.76, -1.78, -1.82, -1.84, 4.12, 4.1, 4.08, -1.22, -1.24, -1.26, -1.52, -1.54, -1.58, -1.62, -1.68, -1.7, -1.72, -1.74, -1.78, -1.8, -1.82, -1.84, -1.86, -1.8800000000000001, 4.2, 4.16, 4.08, -1.68, -1.7, -1.72, -1.74, -1.76, -1.8, -1.82, -1.84, -1.86, -1.8800000000000001, -1.9000000000000001, -1.92, -1.96, -1.98, -2.02, -2.04, -2.06, 4.18, 4.16, 4.12, 4.08, -1.72, -1.74, -1.8, -1.86, -1.9000000000000001, -1.92, -1.94, -1.96, -1.98, -2.06, -2.08, 4.18, 4.16, 4.14, 4.12, 4.1, 4.08, -1.86, -1.8800000000000001, -1.9000000000000001, -1.92, -1.94, -1.96, -2.0, -2.02, -2.06, -2.08, -2.1, -2.14, -2.18, -2.2, -2.22, 4.2, 4.18, 4.16, 4.12, 4.08, -1.86, -1.8800000000000001, -1.92, -1.94, -1.96, -1.98, -2.0, -2.02, -2.04, -2.08, -2.12, -2.16, -2.18, -2.2, -2.22, 4.2, 4.18, 4.16, 4.12, 4.08, -2.0, -2.02, -2.04, -2.06, -2.08, -2.1, -2.12, -2.14, -2.16, -2.18, -2.2, -2.22, -2.24, -2.2600000000000002, -2.2800000000000002, -2.3000000000000003, -2.32, -2.34, -2.36, -2.38, -2.42, -2.44, 4.2, 4.16, 4.12, 4.08, -2.0, -2.02, -2.08, -2.1, -2.12, -2.14, -2.16, -2.18, -2.2, -2.24, -2.2600000000000002, -2.3000000000000003, -2.32, -2.34, -2.4, -2.42, -2.44, 4.2, 4.18, 4.12, 4.08, -2.0, -2.02, -2.04, -2.06, -2.08, -2.12, -2.14, -2.16, -2.18, -2.2, -2.22, -2.2600000000000002, -2.34, -2.36, -2.38, -2.42, -2.46, -2.48, -2.5, -2.52, -2.54, -2.56, 4.2, 4.16, 4.14, 4.1, 4.08, -2.2800000000000002, -2.3000000000000003, -2.32, -2.34, -2.36, -2.38, -2.4, -2.46, -2.5, -2.52, -2.56, -2.58, 4.18, 4.16, 4.12, 4.08, -2.2800000000000002, -2.3000000000000003, -2.34, -2.36, -2.38, -2.4, -2.42, -2.46, -2.48, -2.5, -2.52, -2.54, -2.58, -2.6, 4.2, 4.16, 4.14, 4.12, -2.42, -2.44, -2.46, -2.48, -2.52, -2.54, -2.56, -2.58, -2.6, -2.62, -2.66, -2.68, -2.7, -2.72, 4.2, 4.16, 4.14, 4.12, -2.42, -2.44, -2.46, -2.48, -2.5, -2.52, -2.54, -2.56, -2.6, -2.62, -2.66, -2.68, -2.7, -2.74, -2.56, -2.58, -2.6, -2.62, -2.64, -2.66, -2.68, -2.7, -2.72, -2.74, -2.7800000000000002, -2.8000000000000003, -2.84, 4.22, 4.18, 4.16, -2.56, -2.6, -2.66, -2.68, -2.7, -2.74, -2.7600000000000002, -2.7800000000000002, -2.8000000000000003, -2.82, 4.24, 4.22, 4.2, 4.18, -2.7, -2.72, -2.74, -2.7600000000000002, -2.7800000000000002, -2.8000000000000003, -2.82, -2.84, -2.86, -2.88, -2.9, -2.92, -2.94, -2.96, -2.98, -3.0, -3.02, -3.04, 4.24, 4.22, 4.2, 4.18, 4.16, -2.7, -2.72, -2.7600000000000002, -2.7800000000000002, -2.8000000000000003, -2.84, -2.9, -2.94, -2.96, -3.0, -3.02, 4.24, 4.2, 4.18, -2.84, -2.86, -2.92, -2.94, -3.02, -3.06, -3.1, -3.12, -3.14, -3.18, 4.24, 4.2, 4.18, 4.16, -2.84, -2.86, -2.9, -2.92, -2.94, -2.98, -3.0, -3.02, -3.04, -3.06, -3.08, -3.14, -3.18, 4.2, 4.16, -2.96, -3.0, -3.02, -3.04, -3.08, -3.12, -3.16, -3.18, -3.2, -3.2600000000000002, -3.3000000000000003, -3.3200000000000003, 4.24, 4.22, 4.2, 4.16, -2.98, -3.0, -3.08, -3.12, -3.2, -3.22, -3.24, -3.2600000000000002, -3.2800000000000002, -3.3200000000000003, 4.24, 4.22, 4.2, 4.16, -3.16, -3.18, -3.2600000000000002, -3.3000000000000003, -3.34, -3.36, -3.38, -3.42, -3.44, -3.46, -3.48, -3.52, -3.54, -3.56, -3.58, -3.6, 4.24, 4.16, -3.22, -3.24, -3.2600000000000002, -3.3200000000000003, -3.34, -3.38, -3.4, -3.42, -3.44, -3.5, -3.56, 4.24, 4.22, 4.2, 4.18, 4.16, 4.14, -3.36, -3.4, -3.42, -3.44, -3.48, -3.54, -3.56, -3.62, -3.66, -3.68, 4.24, 4.22, 4.2, 4.18, 4.16, 4.14, -3.38, -3.42, -3.44, -3.48, -3.52, -3.56, -3.58, -3.6, -3.62, -3.66, 4.2, 4.16, 4.14, -3.46, -3.48, -3.5, -3.54, -3.56, -3.58, -3.6, -3.62, -3.64, -3.66, -3.68, -3.7, -3.7800000000000002, 4.22, 4.2, 4.18, 4.16, -3.48, -3.52, -3.54, -3.56, -3.58, -3.6, -3.62, -3.64, -3.68, -3.7, -3.72, -3.74, -3.7600000000000002, -3.7800000000000002, 4.24, 4.22, 4.2, 4.18, -3.6, -3.62, -3.64, -3.66, -3.7, -3.72, -3.74, -3.7800000000000002, -3.8000000000000003, -3.8200000000000003, -3.84, -3.86, -3.9, -3.92, -3.94, -3.96, -3.66, -3.7, -3.74, -3.7600000000000002, -3.7800000000000002, -3.8000000000000003, -3.8200000000000003, -3.88, -3.9, -3.92, -3.94, -3.96, 6.3, 6.26, -3.66, -3.68, -3.7, -3.72, -3.7800000000000002, -3.8200000000000003, -3.84, -3.86, -3.98, -4.0, -4.0200000000000005, -4.0600000000000005, -4.08, -4.1, 6.26, 6.24, -3.74, -3.7600000000000002, -3.7800000000000002, -3.8000000000000003, -3.8200000000000003, -3.88, -3.9, -3.94, -3.96, -3.98, -4.0, -4.04, -4.08, -4.1, 6.32, 6.3, 6.26, 6.24, -3.8000000000000003, -3.8200000000000003, -3.84, -3.86, -3.88, -3.9, -3.96, -3.98, -4.0, -4.0200000000000005, -4.0600000000000005, -4.08, -4.1, 6.32, 6.3, 6.28, 6.26, 6.24, 6.2, -3.94, -3.96, -4.0, -4.04, -4.1, -4.12, -4.14, -4.2, -4.22, -4.24, -4.26, -4.28, 6.32, 6.3, 6.28, 6.24, 6.2, -3.94, -3.96, -4.0, -4.0200000000000005, -4.08, -4.12, -4.14, -4.18, -4.22, -4.24, -4.26, -4.28, -4.3, -4.08, -4.1, -4.12, -4.16, -4.18, -4.22, -4.24, -4.28, -4.3, -4.32, -4.34, -4.36, -4.4, -4.42, -4.08, -4.12, -4.14, -4.16, -4.18, -4.2, -4.22, -4.24, -4.26, -4.28, -4.3, -4.32, -4.36, -4.38, -4.4, -4.42, 4.3, 4.28, 4.24, 4.22, -4.22, -4.24, -4.28, -4.32, -4.36, -4.4, -4.42, -4.44, -4.46, -4.48, -4.5, -4.54, -4.6000000000000005, 4.3, 4.28, 4.26, -4.2, -4.24, -4.28, -4.3, -4.32, -4.34, -4.36, -4.38, -4.42, -4.48, -4.5, -4.5200000000000005, -4.54, -4.58, -4.6000000000000005, -4.62, 4.34, 4.28, 4.24, -4.3, -4.38, -4.42, -4.44, -4.48, -4.5, -4.54, -4.5600000000000005, -4.6000000000000005, -4.62, -4.64, -4.68, -4.7, 4.34, 4.3, 4.28, 4.26, 4.24, -4.3, -4.32, -4.34, -4.36, -4.38, -4.4, -4.42, -4.46, -4.48, -4.5, -4.5200000000000005, -4.5600000000000005, -4.58, -4.62, -4.64, -4.68, -4.7, 4.38, 4.36, 4.34, 4.3, 4.26, -4.44, -4.46, -4.48, -4.5, -4.5200000000000005, -4.54, -4.5600000000000005, -4.62, -4.66, -4.68, -4.72, -4.74, -4.78, -4.8, 4.34, 4.32, 4.3, 4.28, 4.26, -4.44, -4.46, -4.5, -4.54, -4.5600000000000005, -4.6000000000000005, -4.62, -4.72, -4.76, -4.78, -4.8, 4.38, 4.34, 4.32, 4.3, 4.26, -4.64, -4.66, -4.7, -4.72, -4.74, -4.76, -4.78, -4.84, -4.86, -4.88, -4.9, -4.92, 4.38, 4.34, 4.32, 4.3, -4.62, -4.64, -4.66, -4.68, -4.7, -4.76, -4.78, -4.84, -4.94, 4.44, 4.4, 4.36, 4.34, 4.3, -4.72, -4.8, -4.84, -4.88, -4.9, -4.94, -4.96, 4.44, 4.42, 4.4, 4.38, 4.36, 4.34, -4.82, -4.84, -4.86, -4.88, -4.92, -4.94, -4.98, -5.0, -5.0200000000000005, 4.42, 4.4, 4.38, 4.32, 4.3, -4.96, -4.98, -5.0, -5.0200000000000005, 4.42, 4.4, 4.36, 4.34, 4.3, -4.96, -5.0, 4.44, 4.42, 4.38, 4.36, 4.34, 4.32, 4.3, 4.44, 4.42, 4.4, 4.38, 4.36, 4.34, 4.32, 4.44, 4.4, 4.38, 4.34, 4.3, 4.44, 4.4, 4.38, 4.36, 4.44, 4.4, 4.38, 4.36, 4.44, 4.42, 4.44, 4.42, 4.4, 4.38, 4.36, 4.44, 4.38, 4.36, 4.44, 4.4, 4.38, 4.36, 4.38, 4.38, 4.36, 4.38, 4.36, 4.34, 4.32, 4.3, 4.4, 4.38, 4.36, 4.34, 4.32, 4.3, 4.32, 4.44, 4.42, 4.4, 4.38, 4.3, 4.44, 4.36, 4.32, 4.44, 4.42, 4.3, 4.42, 4.4, 4.36, 4.34, 4.44, 4.42, 4.4, 4.38, 4.34, 4.32, 4.44, 4.42, 4.38, 4.34, 4.44, 4.4, 4.36, 4.62, 4.58, 4.62, 4.6000000000000005, 4.62, 4.6000000000000005, 4.58, 4.58, 0.44, 0.42, 0.4, 0.38, 0.32, 0.28, 0.24, -0.1, -0.12, -0.14, -0.18, -0.2, -0.22, -0.24, -0.26, -0.28, 0.42, 0.4, 0.36, 0.34, 0.32, 0.3, 0.28, 0.26, -0.1, -0.14, -0.16, -0.18, -0.2, -0.22, -0.24, -0.26, 0.62, 0.6, 0.56, 0.54, 0.48, 0.46, 0.38, 0.36, 0.3, 0.28, 0.26, -0.12, -0.14, -0.18, -0.2, -0.22, -0.24, -0.26, -0.28, -0.3, -0.34, -0.36, -0.38, -0.42, -0.44, -0.46, -0.48, 0.62, 0.6, 0.58, 0.56, 0.54, 0.52, 0.5, 0.48, 0.46, 0.44, 0.42, 0.4, 0.36, 0.34, 0.3, 0.28, 0.26, -0.14, -0.16, -0.18, -0.2, -0.22, -0.24, -0.26, -0.28, -0.3, -0.32, -0.34, -0.36, -0.38, -0.4, -0.44, -0.48, 0.8200000000000001, 0.72, 0.68, 0.66, 0.62, 0.6, 0.56, 0.52, 0.5, 0.44, 0.42, 0.4, 0.38, 0.36, 0.34, 0.3, 0.28, 0.26, -0.14, -0.2, -0.22, -0.24, -0.26, -0.28, -0.32, -0.36, -0.38, -0.4, -0.42, -0.48, -0.58, -0.62, -0.66, -0.68, -0.76, -0.8, 0.84, 0.8200000000000001, 0.8, 0.78, 0.76, 0.74, 0.72, 0.66, 0.64, 0.62, 0.56, 0.54, -0.34, -0.36, -0.38, -0.4, -0.44, -0.48, -0.5, -0.52, -0.54, -0.56, -0.62, -0.64, -0.66, -0.68, -0.72, -0.76, -0.78, -0.8, 0.8200000000000001, 0.74, 0.72, 0.7000000000000001, 0.62, 0.58, 0.56, 0.54, -0.36, -0.38, -0.42, -0.44, -0.52, -0.54, -0.56, -0.58, -0.62, -0.64, -0.66, -0.68, -0.7000000000000001, -0.72, -0.76, -0.78, -0.8, -0.8200000000000001, -0.6, -0.62, -0.64, -0.66, -0.7000000000000001, -0.72, -0.74, -0.76, -0.8, -0.8200000000000001, -0.58, -0.62, -0.66, -0.7000000000000001, -0.72, -0.76, -0.78, -0.8, -0.8200000000000001, -1.1400000000000001, -1.16, -1.2, 1.16, 1.1400000000000001, -1.12, -1.1400000000000001, -1.16, -1.2, -1.22, 1.18, 1.1400000000000001, -1.12, -1.1400000000000001, -1.2, -1.22, 1.18, 1.16, -1.1400000000000001, -1.16, -1.2, -1.22, -1.52, -1.54, -1.58, -1.52, -1.54, -1.58, -1.52, -1.54, -1.56, -1.6, -1.62, -1.6600000000000001, -1.54, -1.56, -1.58, -1.6, -1.6400000000000001, -1.6600000000000001, 1.54, 1.52, 1.5, -1.54, -1.56, -1.58, -1.6, -1.62, -1.6600000000000001, -1.72, -1.74, -1.76, -1.78, -1.8, -1.82, -1.84, 1.54, 1.52, 1.5, -1.68, -1.7, -1.74, -1.76, -1.78, -1.8, -1.82, -1.84, -1.86, 1.6600000000000001, 1.6400000000000001, 1.54, 1.5, -1.68, -1.7, -1.74, -1.76, -1.78, -1.8, -1.9000000000000001, -1.92, 1.68, 1.6600000000000001, 1.6400000000000001, -1.82, -1.9000000000000001, -1.92, -1.94, -1.96, -1.98, 1.6400000000000001, -1.82, -1.84, -1.86, -1.9000000000000001, -1.92, -1.96, -1.98, -2.0, 1.68, 1.6600000000000001, 1.6400000000000001, -1.92, -1.98, -2.02, -2.04, -2.06, -2.08, -2.1, -2.12, -2.14, -2.18, 1.68, 1.6600000000000001, 1.6400000000000001, -1.94, -1.96, -1.98, -2.02, -2.06, -2.08, -2.1, -2.12, -2.16, -2.18, -2.0, -2.04, -2.06, -2.08, -2.1, -2.12, -2.14, -2.18, -2.2, -2.22, -2.24, -2.2800000000000002, -2.3000000000000003, -2.32, -2.04, -2.06, -2.08, -2.1, -2.12, -2.16, -2.2, -2.24, -2.2600000000000002, -2.2800000000000002, -2.3000000000000003, -2.1, -2.12, -2.14, -2.16, -2.18, -2.2, -2.2600000000000002, -2.2800000000000002, -2.3000000000000003, -2.34, -2.36, -2.4, -2.42, -2.44, -2.48, -2.5, -2.1, -2.18, -2.2, -2.22, -2.24, -2.2600000000000002, -2.2800000000000002, -2.3000000000000003, -2.38, -2.46, -2.48, -2.5, -2.12, -2.14, -2.16, -2.18, -2.22, -2.24, -2.2600000000000002, -2.2800000000000002, -2.3000000000000003, -2.34, -2.36, -2.38, -2.4, -2.44, -2.48]
  out "x":dbl[](array[numeric])=[-2.06, -2.06, -2.06, -2.06, -2.04, -2.04, -2.04, -2.04, -2.02, -2.02, -2.02, -2.02, -2.0, -2.0, -2.0, -2.0, -2.0, -1.98, -1.96, -1.96, -1.96, -1.94, -1.94, -1.94, -1.94, -1.92, -1.92, -1.92, -1.92, -1.9000000000000001, -1.9000000000000001, -1.8800000000000001, -1.8800000000000001, -1.86, -1.86, -1.86, -1.86, -1.84, -1.84, -1.84, -1.82, -1.82, -1.82, -1.82, -1.82, -1.82, -1.82, -1.82, -1.8, -1.8, -1.8, -1.8, -1.8, -1.8, -1.8, -1.8, -1.8, -1.78, -1.78, -1.78, -1.78, -1.78, -1.78, -1.78, -1.78, -1.76, -1.76, -1.76, -1.74, -1.74, -1.74, -1.74, -1.74, -1.74, -1.74, -1.74, -1.74, -1.74, -1.74, -1.74, -1.74, -1.74, -1.74, -1.72, -1.72, -1.72, -1.72, -1.72, -1.72, -1.72, -1.72, -1.72, -1.72, -1.7, -1.7, -1.7, -1.7, -1.7, -1.7, -1.7, -1.7, -1.7, -1.7, -1.7, -1.7, -1.7, -1.7, -1.7, -1.7, -1.7, -1.68, -1.68, -1.68, -1.68, -1.68, -1.68, -1.6600000000000001, -1.6600000000000001, -1.6600000000000001, -1.6600000000000001, -1.6600000000000001, -1.6600000000000001, -1.6600000000000001, -1.6600000000000001, -1.6600000000000001, -1.6600000000000001, -1.6600000000000001, -1.6400000000000001, -1.6400000000000001, -1.6400000000000001, -1.6400000000000001, -1.6400000000000001, -1.6400000000000001, -1.62, -1.62, -1.62, -1.62, -1.62, -1.62, -1.62, -1.6, -1.6, -1.6, -1.58, -1.58, -1.58, -1.56, -1.56, -1.56, -1.54, -1.54, -1.54, -1.52, -1.52, -1.52, -1.52, -1.52, -1.52, -1.52, -1.52, -1.52, -1.5, -1.5, -1.5, -1.5, -1.5, -1.5, -1.48, -1.48, -1.48, -1.48, -1.48, -1.48, -1.48, -1.48, -1.48, -1.48, -1.48, -1.48, -1.48, -1.46, -1.46, -1.46, -1.46, -1.46, -1.46, -1.46, -1.46, -1.46, -1.46, -1.46, -1.46, -1.46, -1.46, -1.46, -1.46, -1.44, -1.44, -1.44, -1.44, -1.44, -1.44, -1.44, -1.44, -1.44, -1.44, -1.44, -1.44, -1.44, -1.44, -1.44, -1.44, -1.42, -1.42, -1.42, -1.42, -1.42, -1.42, -1.42, -1.42, -1.42, -1.42, -1.42, -1.42, -1.42, -1.42, -1.42, -1.42, -1.42, -1.42, -1.42, -1.42, -1.4000000000000001, -1.4000000000000001, -1.4000000000000001, -1.4000000000000001, -1.4000000000000001, -1.4000000000000001, -1.4000000000000001, -1.4000000000000001, -1.4000000000000001, -1.4000000000000001, -1.4000000000000001, -1.4000000000000001, -1.4000000000000001, -1.4000000000000001, -1.4000000000000001, -1.4000000000000001, -1.4000000000000001, -1.4000000000000001, -1.4000000000000001, -1.4000000000000001, -1.3800000000000001, -1.3800000000000001, -1.3800000000000001, -1.3800000000000001, -1.3800000000000001, -1.3800000000000001, -1.3800000000000001, -1.3800000000000001, -1.3800000000000001, -1.3800000000000001, -1.3800000000000001, -1.3800000000000001, -1.3800000000000001, -1.3800000000000001, -1.3800000000000001, -1.36, -1.36, -1.36, -1.36, -1.36, -1.36, -1.36, -1.36, -1.36, -1.36, -1.36, -1.36, -1.36, -1.36, -1.36, -1.36, -1.36, -1.36, -1.36, -1.36, -1.36, -1.34, -1.34, -1.34, -1.34, -1.34, -1.34, -1.34, -1.34, -1.34, -1.34, -1.34, -1.34, -1.34, -1.34, -1.34, -1.34, -1.34, -1.34, -1.34, -1.34, -1.32, -1.32, -1.32, -1.32, -1.32, -1.32, -1.32, -1.32, -1.32, -1.32, -1.32, -1.32, -1.32, -1.32, -1.32, -1.32, -1.32, -1.32, -1.32, -1.32, -1.32, -1.32, -1.32, -1.32, -1.32, -1.32, -1.32, -1.3, -1.3, -1.3, -1.3, -1.3, -1.3, -1.3, -1.3, -1.3, -1.3, -1.3, -1.3, -1.3, -1.3, -1.3, -1.3, -1.3, -1.3, -1.3, -1.3, -1.3, -1.28, -1.28, -1.28, -1.28, -1.28, -1.28, -1.28, -1.28, -1.28, -1.28, -1.28, -1.28, -1.28, -1.28, -1.28, -1.28, -1.28, -1.28, -1.28, -1.28, -1.28, -1.28, -1.28, -1.28, -1.28, -1.28, -1.26, -1.26, -1.26, -1.26, -1.26, -1.26, -1.26, -1.26, -1.26, -1.26, -1.26, -1.26, -1.26, -1.26, -1.26, -1.26, -1.26, -1.24, -1.24, -1.24, -1.24, -1.24, -1.24, -1.24, -1.24, -1.24, -1.24, -1.24, -1.24, -1.24, -1.24, -1.24, -1.24, -1.24, -1.24, -1.22, -1.22, -1.22, -1.22, -1.22, -1.22, -1.22, -1.22, -1.22, -1.22, -1.22, -1.22, -1.22, -1.22, -1.22, -1.22, -1.22, -1.22, -1.2, -1.2, -1.2, -1.2, -1.2, -1.2, -1.2, -1.2, -1.2, -1.2, -1.2, -1.2, -1.2, -1.2, -1.2, -1.2, -1.2, -1.2, -1.18, -1.18, -1.18, -1.18, -1.18, -1.18, -1.18, -1.18, -1.18, -1.18, -1.18, -1.18, -1.18, -1.16, -1.16, -1.16, -1.16, -1.16, -1.16, -1.16, -1.16, -1.16, -1.16, -1.16, -1.16, -1.16, -1.1400000000000001, -1.1400000000000001, -1.1400000000000001, -1.1400000000000001, -1.1400000000000001, -1.1400000000000001, -1.1400000000000001, -1.1400000000000001, -1.1400000000000001, -1.1400000000000001, -1.1400000000000001, -1.1400000000000001, -1.1400000000000001, -1.1400000000000001, -1.1400000000000001, -1.1400000000000001, -1.1400000000000001, -1.1400000000000001, -1.1400000000000001, -1.1400000000000001, -1.1400000000000001, -1.1400000000000001, -1.12, -1.12, -1.12, -1.12, -1.12, -1.12, -1.12, -1.12, -1.12, -1.12, -1.12, -1.12, -1.12, -1.12, -1.12, -1.12, -1.1, -1.1, -1.1, -1.1, -1.1, -1.1, -1.1, -1.1, -1.1, -1.1, -1.1, -1.1, -1.1, -1.08, -1.08, -1.08, -1.08, -1.08, -1.08, -1.08, -1.08, -1.08, -1.08, -1.08, -1.08, -1.08, -1.08, -1.08, -1.08, -1.08, -1.06, -1.06, -1.06, -1.06, -1.06, -1.06, -1.06, -1.06, -1.06, -1.06, -1.06, -1.06, -1.06, -1.06, -1.04, -1.04, -1.04, -1.04, -1.04, -1.04, -1.04, -1.04, -1.04, -1.04, -1.04, -1.04, -1.04, -1.04, -1.02, -1.02, -1.02, -1.02, -1.02, -1.02, -1.02, -1.02, -1.02, -1.02, -1.02, -1.02, -1.02, -1.02, -1.02, -1.02, -1.02, -1.02, -1.02, -1.02, -1.0, -1.0, -1.0, -1.0, -1.0, -1.0, -1.0, -1.0, -1.0, -1.0, -1.0, -1.0, -1.0, -0.98, -0.98, -0.98, -0.98, -0.98, -0.98, -0.98, -0.98, -0.98, -0.98, -0.98, -0.98, -0.98, -0.98, -0.98, -0.98, -0.96, -0.96, -0.96, -0.96, -0.96, -0.96, -0.96, -0.96, -0.96, -0.96, -0.96, -0.96, -0.96, -0.96, -0.96, -0.96, -0.9400000000000001, -0.9400000000000001, -0.9400000000000001, -0.9400000000000001, -0.9400000000000001, -0.9400000000000001, -0.9400000000000001, -0.9400000000000001, -0.9400000000000001, -0.9400000000000001, -0.9400000000000001, -0.9400000000000001, -0.9400000000000001, -0.9400000000000001, -0.9400000000000001, -0.9400000000000001, -0.92, -0.92, -0.92, -0.92, -0.92, -0.92, -0.92, -0.92, -0.92, -0.92, -0.92, -0.92, -0.92, -0.92, -0.92, -0.92, -0.92, -0.92, -0.9, -0.9, -0.9, -0.9, -0.9, -0.9, -0.9, -0.9, -0.9, -0.9, -0.9, -0.9, -0.9, -0.9, -0.9, -0.9, -0.9, -0.9, -0.9, -0.9, -0.88, -0.88, -0.88, -0.88, -0.88, -0.88, -0.88, -0.88, -0.88, -0.88, -0.88, -0.88, -0.86, -0.86, -0.86, -0.86, -0.86, -0.86, -0.86, -0.86, -0.86, -0.86, -0.86, -0.86, -0.86, -0.86, -0.86, -0.86, -0.84, -0.84, -0.84, -0.84, -0.84, -0.84, -0.84, -0.84, -0.84, -0.84, -0.84, -0.84, -0.84, -0.84, -0.84, -0.84, -0.8200000000000001, -0.8200000000000001, -0.8200000000000001, -0.8200000000000001, -0.8200000000000001, -0.8200000000000001, -0.8200000000000001, -0.8200000000000001, -0.8200000000000001, -0.8200000000000001, -0.8200000000000001, -0.8200000000000001, -0.8200000000000001, -0.8200000000000001, -0.8200000000000001, -0.8200000000000001, -0.8200000000000001, -0.8, -0.8, -0.8, -0.8, -0.8, -0.8, -0.8, -0.8, -0.8, -0.8, -0.8, -0.8, -0.8, -0.8, -0.8, -0.8, -0.8, -0.8, -0.78, -0.78, -0.78, -0.78, -0.78, -0.78, -0.78, -0.78, -0.78, -0.78, -0.78, -0.78, -0.78, -0.78, -0.78, -0.78, -0.78, -0.78, -0.76, -0.76, -0.76, -0.76, -0.76, -0.76, -0.76, -0.76, -0.76, -0.76, -0.76, -0.76, -0.76, -0.76, -0.74, -0.74, -0.74, -0.74, -0.74, -0.74, -0.74, -0.74, -0.74, -0.74, -0.74, -0.74, -0.74, -0.74, -0.74, -0.74, -0.72, -0.72, -0.72, -0.72, -0.72, -0.72, -0.72, -0.72, -0.72, -0.72, -0.72, -0.72, -0.72, -0.72, -0.72, -0.72, -0.72, -0.7000000000000001, -0.7000000000000001, -0.7000000000000001, -0.7000000000000001, -0.7000000000000001, -0.7000000000000001, -0.7000000000000001, -0.7000000000000001, -0.7000000000000001, -0.7000000000000001, -0.7000000000000001, -0.7000000000000001, -0.7000000000000001, -0.7000000000000001, -0.7000000000000001, -0.7000000000000001, -0.7000000000000001, -0.7000000000000001, -0.7000000000000001, -0.68, -0.68, -0.68, -0.68, -0.68, -0.68, -0.68, -0.68, -0.68, -0.68, -0.68, -0.68, -0.68, -0.68, -0.68, -0.68, -0.66, -0.66, -0.66, -0.66, -0.66, -0.66, -0.66, -0.66, -0.66, -0.66, -0.66, -0.66, -0.66, -0.66, -0.66, -0.66, -0.66, -0.66, -0.66, -0.66, -0.66, -0.66, -0.64, -0.64, -0.64, -0.64, -0.64, -0.64, -0.64, -0.64, -0.64, -0.64, -0.64, -0.64, -0.64, -0.64, -0.64, -0.64, -0.64, -0.64, -0.64, -0.62, -0.62, -0.62, -0.62, -0.62, -0.62, -0.62, -0.62, -0.62, -0.62, -0.62, -0.62, -0.62, -0.62, -0.62, -0.62, -0.6, -0.6, -0.6, -0.6, -0.6, -0.6, -0.6, -0.6, -0.6, -0.6, -0.6, -0.6, -0.6, -0.6, -0.6, -0.6, -0.6, -0.58, -0.58, -0.58, -0.58, -0.58, -0.58, -0.58, -0.58, -0.58, -0.58, -0.58, -0.58, -0.58, -0.56, -0.56, -0.56, -0.56, -0.56, -0.56, -0.56, -0.56, -0.56, -0.56, -0.56, -0.56, -0.54, -0.54, -0.54, -0.54, -0.54, -0.54, -0.54, -0.54, -0.54, -0.54, -0.54, -0.54, -0.54, -0.54, -0.54, -0.52, -0.52, -0.52, -0.52, -0.52, -0.52, -0.52, -0.52, -0.52, -0.5, -0.5, -0.5, -0.5, -0.5, -0.5, -0.5, -0.48, -0.48, -0.48, -0.48, -0.48, -0.48, -0.48, -0.46, -0.46, -0.46, -0.46, -0.46, -0.46, -0.46, -0.44, -0.44, -0.44, -0.44, -0.44, -0.42, -0.42, -0.42, -0.42, -0.4, -0.4, -0.4, -0.4, -0.38, -0.38, -0.36, -0.36, -0.36, -0.36, -0.36, -0.34, -0.34, -0.34, -0.32, -0.32, -0.32, -0.32, -0.3, -0.28, -0.28, -0.26, -0.26, -0.26, -0.26, -0.26, -0.24, -0.24, -0.24, -0.24, -0.24, -0.24, -0.22, -0.2, -0.2, -0.2, -0.2, -0.2, -0.18, -0.18, -0.18, -0.16, -0.16, -0.16, -0.14, -0.14, -0.14, -0.14, -0.12, -0.12, -0.12, -0.12, -0.12, -0.12, -0.1, -0.1, -0.1, -0.1, -0.08, -0.08, -0.08, 0.32, 0.32, 0.34, 0.34, 0.36, 0.36, 0.36, 0.38, 1.62, 1.62, 1.62, 1.62, 1.62, 1.62, 1.62, 1.62, 1.62, 1.62, 1.62, 1.62, 1.62, 1.62, 1.62, 1.62, 1.6400000000000001, 1.6400000000000001, 1.6400000000000001, 1.6400000000000001, 1.6400000000000001, 1.6400000000000001, 1.6400000000000001, 1.6400000000000001, 1.6400000000000001, 1.6400000000000001, 1.6400000000000001, 1.6400000000000001, 1.6400000000000001, 1.6400000000000001, 1.6400000000000001, 1.6400000000000001, 1.6600000000000001, 1.6600000000000001, 1.6600000000000001, 1.6600000000000001, 1.6600000000000001, 1.6600000000000001, 1.6600000000000001, 1.6600000000000001, 1.6600000000000001, 1.6600000000000001, 1.6600000000000001, 1.6600000000000001, 1.6600000000000001, 1.6600000000000001, 1.6600000000000001, 1.6600000000000001, 1.6600000000000001, 1.6600000000000001, 1.6600000000000001, 1.6600000000000001, 1.6600000000000001, 1.6600000000000001, 1.6600000000000001, 1.6600000000000001, 1.6600000000000001, 1.6600000000000001, 1.6600000000000001, 1.68, 1.68, 1.68, 1.68, 1.68, 1.68, 1.68, 1.68, 1.68, 1.68, 1.68, 1.68, 1.68, 1.68, 1.68, 1.68, 1.68, 1.68, 1.68, 1.68, 1.68, 1.68, 1.68, 1.68, 1.68, 1.68, 1.68, 1.68, 1.68, 1.68, 1.68, 1.68, 1.68, 1.7, 1.7, 1.7, 1.7, 1.7, 1.7, 1.7, 1.7, 1.7, 1.7, 1.7, 1.7, 1.7, 1.7, 1.7, 1.7, 1.7, 1.7, 1.7, 1.7, 1.7, 1.7, 1.7, 1.7, 1.7, 1.7, 1.7, 1.7, 1.7, 1.7, 1.7, 1.7, 1.7, 1.7, 1.7, 1.7, 1.72, 1.72, 1.72, 1.72, 1.72, 1.72, 1.72, 1.72, 1.72, 1.72, 1.72, 1.72, 1.72, 1.72, 1.72, 1.72, 1.72, 1.72, 1.72, 1.72, 1.72, 1.72, 1.72, 1.72, 1.72, 1.72, 1.72, 1.72, 1.72, 1.72, 1.74, 1.74, 1.74, 1.74, 1.74, 1.74, 1.74, 1.74, 1.74, 1.74, 1.74, 1.74, 1.74, 1.74, 1.74, 1.74, 1.74, 1.74, 1.74, 1.74, 1.74, 1.74, 1.74, 1.74, 1.74, 1.74, 1.76, 1.76, 1.76, 1.76, 1.76, 1.76, 1.76, 1.76, 1.76, 1.76, 1.78, 1.78, 1.78, 1.78, 1.78, 1.78, 1.78, 1.78, 1.78, 1.84, 1.84, 1.84, 1.86, 1.86, 1.86, 1.86, 1.86, 1.86, 1.86, 1.8800000000000001, 1.8800000000000001, 1.8800000000000001, 1.8800000000000001, 1.8800000000000001, 1.8800000000000001, 1.9000000000000001, 1.9000000000000001, 1.9000000000000001, 1.9000000000000001, 1.9000000000000001, 1.9000000000000001, 2.04, 2.04, 2.04, 2.06, 2.06, 2.06, 2.08, 2.08, 2.08, 2.08, 2.08, 2.08, 2.1, 2.1, 2.1, 2.1, 2.1, 2.1, 2.12, 2.12, 2.12, 2.12, 2.12, 2.12, 2.12, 2.12, 2.12, 2.12, 2.12, 2.12, 2.12, 2.12, 2.12, 2.12, 2.14, 2.14, 2.14, 2.14, 2.14, 2.14, 2.14, 2.14, 2.14, 2.14, 2.14, 2.14, 2.16, 2.16, 2.16, 2.16, 2.16, 2.16, 2.16, 2.16, 2.16, 2.16, 2.16, 2.16, 2.18, 2.18, 2.18, 2.18, 2.18, 2.18, 2.18, 2.18, 2.18, 2.2, 2.2, 2.2, 2.2, 2.2, 2.2, 2.2, 2.2, 2.2, 2.22, 2.22, 2.22, 2.22, 2.22, 2.22, 2.22, 2.22, 2.22, 2.22, 2.22, 2.22, 2.22, 2.24, 2.24, 2.24, 2.24, 2.24, 2.24, 2.24, 2.24, 2.24, 2.24, 2.24, 2.24, 2.24, 2.2600000000000002, 2.2600000000000002, 2.2600000000000002, 2.2600000000000002, 2.2600000000000002, 2.2600000000000002, 2.2600000000000002, 2.2600000000000002, 2.2600000000000002, 2.2600000000000002, 2.2600000000000002, 2.2600000000000002, 2.2600000000000002, 2.2600000000000002, 2.2800000000000002, 2.2800000000000002, 2.2800000000000002, 2.2800000000000002, 2.2800000000000002, 2.2800000000000002, 2.2800000000000002, 2.2800000000000002, 2.2800000000000002, 2.2800000000000002, 2.2800000000000002, 2.3000000000000003, 2.3000000000000003, 2.3000000000000003, 2.3000000000000003, 2.3000000000000003, 2.3000000000000003, 2.3000000000000003, 2.3000000000000003, 2.3000000000000003, 2.3000000000000003, 2.3000000000000003, 2.3000000000000003, 2.3000000000000003, 2.3000000000000003, 2.3000000000000003, 2.3000000000000003, 2.32, 2.32, 2.32, 2.32, 2.32, 2.32, 2.32, 2.32, 2.32, 2.32, 2.32, 2.32, 2.34, 2.34, 2.34, 2.34, 2.34, 2.34, 2.34, 2.34, 2.34, 2.34, 2.34, 2.34, 2.34, 2.34, 2.34]
  out "r":dbl[](array[numeric])=[-4.6555, -4.935824427641934, -5.2430046330557945, -5.581538421297181, -5.956978730736188, -6.376262963548993, -6.848173849885621, -7.3839975089910626, -7.9984847100349565, -8.711291873800976, -9.549206492141174, -10.549704845388673, -11.766875707952016, -13.281774570932784, -15.221624936294774, -17.79815033646731, -21.39170207506112, -26.760884248621494, -35.66835875277913, -53.36351887551581, -105.63868975677755, -4880.214687241169, 110.4221450101935, 54.55969083607183, 36.20050875601431, 27.06064856420524, 21.583909481852253, 17.931933528233145, 15.32018130844496, 13.357468347457555, 11.82689587838567, 10.598514680927435, 9.589722854776836, 8.745501286784753, 8.0277867617425, 7.409406661367354, 6.870443364939505, 6.395963884688509, 5.974551847557845, 5.597329415527146, 5.257288430183145, 4.948822433014104, 4.667392532060661]
  out "rout":dbl[](array[numeric])=[-6.324751398276457, -6.568080531230865, -6.837975211649557, -7.138909764277184, -7.47641368355318, -7.857400977550082, -8.290631051860542, -8.787366797122555, -9.362335883352985, -10.035171802646554, -10.83263933752883, -11.792192335500603, -12.967897480282396, -14.440788588805296, -16.338067988575105, -18.871438629257682, -22.421231923965998, -27.746032879781435, -36.6084852202519, -54.257965101709786, -106.48678170148416, -4881.015736203275, 111.26816948556541, 55.45209977508024, 37.13862744103356, 28.043818185442433, 22.611488312177844, 19.00329796919853, 16.434726812975573, 14.514610225881459, 13.026069995343686, 11.839178051339472, 10.871354147440517, 10.067601244388326, 9.389878546115288, 8.8110361326976, 8.311179303489036, 7.875398163251261, 7.492299562567518, 7.153028984337258, 6.8506016616375085, 6.5794345780109555, 6.335012320401018]
  out "rin":dbl[](array[numeric])=[-3.8555, -4.135824427641934, -4.443004633055795, -4.781538421297181, -5.1569787307361885, -5.576262963548993, -6.048173849885621, -6.583997508991063, -7.198484710034957, -7.911291873800976, -8.749206492141173, -9.749704845388672, -10.966875707952015, -12.481774570932783, -14.421624936294773, -16.998150336467308, -20.591702075061118, -25.960884248621493, -34.86835875277913, -52.56351887551581, -104.83868975677755, -4879.414687241168, 109.6221450101935, 53.75969083607183, 35.40050875601431, 26.26064856420524, 20.783909481852252, 17.131933528233144, 14.52018130844496, 12.557468347457554, 11.02689587838567, 9.798514680927434, 8.789722854776835, 7.945501286784753, 7.227786761742499, 6.6094066613673546, 6.070443364939505, 5.595963884688509, 5.174551847557845, 4.797329415527146, 4.457288430183145, 4.148822433014105, 3.867392532060661]
  out "XY Graph":cluster{"Y":dbl[], "Y":dbl[]}[](graph)=[{"Y"=array[1490 elements], "Y"=array[1490 elements]}, {"Y"=[-0.5, -0.5, -0.5, -0.6000000000000001, -0.6000000000000001, -0.6000000000000001, -0.6000000000000001, -0.6000000000000001, -0.6000000000000001, -0.6000000000000001, -0.7000000000000001, -0.7000000000000001, -0.7000000000000001, -0.7000000000000001, -0.7000000000000001, -0.7000000000000001, -0.7000000000000001, -0.8, -0.8, -0.8, -0.8, -0.8, -0.8, -0.8, -0.8, -0.9, -0.9, -0.9, -0.9, -0.9, -0.9, -0.9, -1.0, -1.0, -1.0, -1.0, -1.0, -1.0, -1.0, -1.0, -1.1, -1.1, -1.1, -1.1, -1.1, -1.1, -1.1, -1.2000000000000002, -1.2000000000000002, -1.2000000000000002, -1.2000000000000002, -1.2000000000000002, -1.2000000000000002, -1.3, -1.3, -1.3, -1.3, -1.3, -1.3, -1.3, -1.3, -1.4000000000000001, -1.4000000000000001, -1.4000000000000001, -1.4000000000000001, -1.4000000000000001, -1.4000000000000001, -1.4000000000000001, -1.4000000000000001, -1.4000000000000001, -1.4000000000000001, -1.5, -1.5, -1.5, -1.5, -1.5, -1.5, -1.6, -1.6, -1.6, -1.7000000000000002, -1.7000000000000002, -1.7000000000000002, -1.7000000000000002, -1.7000000000000002, -1.7000000000000002, -1.8, -1.8, -1.8], "Y"=[-4.800000000000001, -4.9, -5.0, -4.4, -4.5, -4.6000000000000005, -4.7, -4.800000000000001, -4.9, -5.0, -4.1000000000000005, -4.2, -4.3, -4.4, -4.5, -4.6000000000000005, -4.7, -3.7, -3.8000000000000003, -3.9000000000000004, -4.0, -4.1000000000000005, -4.2, -4.3, -4.4, -3.5, -3.6, -3.7, -3.8000000000000003, -3.9000000000000004, -4.0, -4.1000000000000005, -3.0, -3.1, -3.2, -3.3000000000000003, -3.4000000000000004, -3.5, -3.6, -3.7, -2.7, -2.8000000000000003, -2.9000000000000004, -3.0, -3.1, -3.2, -3.3000000000000003, -2.3000000000000003, -2.4000000000000004, -2.5, -2.6, -2.7, -2.8000000000000003, -1.9000000000000001, -2.0, -2.1, -2.2, -2.3000000000000003, -2.4000000000000004, -2.5, -2.6, -1.2000000000000002, -1.3, -1.5, -1.6, -1.7000000000000002, -1.8, -1.9000000000000001, -2.0, -2.1, -2.2, -1.1, -1.2000000000000002, -1.4000000000000001, -1.5, -1.6, -1.7000000000000002, -0.8, -0.9, -1.1, -0.4, -0.5, -0.6000000000000001, -0.7000000000000001, -0.8, -0.9, -0.2, -0.30000000000000004, -0.4]}, {"Y"=[2.3000000000000003, 2.3000000000000003, 2.3000000000000003, 2.3000000000000003, 2.3000000000000003, 2.3000000000000003, 2.2, 2.2, 2.2, 2.2, 2.2, 2.2, 2.2, 2.2, 2.2, 2.1, 2.1, 2.1, 2.1, 2.1, 2.1, 2.0, 2.0, 1.9000000000000001, 1.9000000000000001, 1.8, 1.8, 1.8, 1.8, 1.8, 1.7000000000000002, 1.7000000000000002, 1.7000000000000002, 1.7000000000000002, 1.7000000000000002, 1.7000000000000002, 1.7000000000000002, 1.7000000000000002, 1.7000000000000002, 1.7000000000000002, 1.7000000000000002, 1.7000000000000002, 1.7000000000000002, 1.7000000000000002, 1.6, 1.6, 1.6, 1.6, 1.6, 1.6], "Y"=[-2.0, -2.1, -2.2, -2.3000000000000003, -2.4000000000000004, -2.5, 1.7000000000000002, 1.6, 1.5, -1.7000000000000002, -1.8, -1.9000000000000001, -2.0, -2.1, -2.2, 1.5, -1.5, -1.6, -1.7000000000000002, -1.8, -1.9000000000000001, -1.5, -1.6, -1.1, -1.2000000000000002, -0.6000000000000001, -0.7000000000000001, -0.8, -1.1, -1.2000000000000002, 0.8, 0.7000000000000001, 0.6000000000000001, 0.5, 0.4, 0.30000000000000004, -0.1, -0.2, -0.30000000000000004, -0.4, -0.5, -0.6000000000000001, -0.7000000000000001, -0.8, 0.4, 0.30000000000000004, 0.2, -0.1, -0.2, -0.30000000000000004]}, {"Y"=array[630 elements], "Y"=array[630 elements]}, {"Y"=array[630 elements], "Y"=array[630 elements]}, {"Y"=array[630 elements], "Y"=array[630 elements]}, {"Y"=[7.816394639851724, 7.319850750911751, 6.817348511778361, 6.318251688313182, 5.827348177464875, 5.357007078148591, 4.915309928811384, 4.506393003662533, 4.139164703638908, 3.8204251317486726, 3.553125525255061, 3.3414092817759076, 3.162481577170565, 2.974816018164504, 2.7663181983145737, 2.5568038965593267, 2.346281212841328, 2.137110915736132, 1.9078677144083886, 1.6966257339926898, 1.4727897553614842, 1.267204576151037, 1.056195582801043, 0.8646221231359237, 0.6899396920978118, 0.5334627663349991, 0.38672572067820976, 0.24339724215034841, 0.1456482869244913, 0.07690190270719764, 0.07504130918645387, 0.15056146198230025, 0.2713581716204574, 0.48389367093431557, 0.7635759918697156, 1.093879975509565, 1.4677637527600913, 1.8763550195382899, 2.3153426039393317, 2.771874137881789, 3.231370665823273, 3.6509816858036017, 4.070592705783319, 4.490203725763379, 4.909814747693659, 5.329425767673296, 5.749036787653171, 6.221881697921817, 6.699225266787154, 7.177159239828125, 7.6557860912435425, 8.133025174001979, 8.628550403441674, 9.124008743619601, 9.613616845908991, 10.086525367124885, 10.584289234819206, 11.080641638604668, 11.582849558630004, 12.062121491179392, 12.540326896884341, 13.046909151428244, 13.554940980687112, 14.041806127624989, 14.542723876848166, 15.020985202042274, 15.505141607780933, 15.99311310838169, 16.493060444282225, 16.97550279588125, 17.462933231924865, 17.955771199982937, 18.449162785063116, 18.938182613989092, 19.427658560604403, 19.922519917978587, 20.42188019851678, 20.931285131759044, 21.43952238396465, 21.956510957892004, 22.463501299867655], "Y"=[-11.502422251196494, -11.568849855643048, -11.569869129213243, -11.520860138841421, -11.405170845617462, -11.226259490137743, -10.988893406280077, -10.696478505477039, -10.350566631066288, -9.958991100165163, -9.530708293774902, -9.076698909741534, -8.606503294262685, -8.139646975484823, -7.675177371218184, -7.212748738665048, -6.758736023816151, -6.300936320923626, -5.855089012523531, -5.394632350417117, -4.92904856027104, -4.473226890410778, -4.019265331616374, -3.5554085848815493, -3.086532078701303, -2.6094805590208754, -2.1284651391769147, -1.6493875550133497, -1.154198294196969, -0.6553479932436498, -0.14705148394533343, 0.3495082078877353, 0.840275199270352, 1.2950552074773085, 1.7139922024325969, 2.091455354026735, 2.424471695783147, 2.7142412798840154, 2.9593516326772193, 3.1677381667356266, 3.373124974874619, 3.571397041456308, 3.76966910803638, 3.9679411746171946, 4.166213251006239, 4.364485317587152, 4.562757384167902, 4.728902132967184, 4.893725317609852, 5.06325165554511, 5.223036909273246, 5.382011198665163, 5.546222380223215, 5.708907308255361, 5.868935992202126, 6.031944130466162, 6.194471477185138, 6.35598661708894, 6.520343533121731, 6.686404463094906, 6.851993294039719, 7.0204856344182245, 7.184294420682817, 7.35241936258849, 7.5192717503812485, 7.678685140450257, 7.845257459374583, 8.007859664044247, 8.172687410639393, 8.329345654397303, 8.483897842226659, 8.635186977264295, 8.778973143211905, 8.910395437670521, 9.02767533114414, 9.127472540585499, 9.208969224478702, 9.27032570434919, 9.307930968543975, 9.319536747877331, 9.309462952310396]}, {"Y"=[-0.23471911221011726, 0.13856315350095594, 0.9014268763793528, 1.5953000420032126, 2.2688338651612834, 2.951352305493015, 3.615197876285664, 4.280325955640375, 4.894222310601533, 5.366855054082828, 5.782862753334636, 6.202473773320374, 6.6220847932977245, 7.041695777086183, 7.461306835206849, 7.88091785518761, 8.502886088631676, 8.98553476608143, 9.447680181790954, 9.95915434390564, 10.438942410664858, 10.918927284847708, 11.419277073808205, 11.917117653408722, 12.378234679666264, 12.880166216346565, 13.379689601946069, 13.873087643567787, 14.34458204422441, 14.824199305123472, 15.324289973918983, 15.846999727487516, 16.31854769679266, 16.824992860827617, 17.325551717055784, 17.786641991392493, 18.288125455255955, 18.781715131857183, 19.289545148899034, 19.784042284874406, 20.287274061456333, 20.804143240880112, 21.33187890403804, 21.863695838788075, 22.406357373710716], "Y"=[3.1368560180005147, 3.6479708862567946, 4.078023402463962, 4.40065915491611, 4.648987727964748, 4.817220667355426, 4.928174290964523, 4.9727637478653435, 5.0158971484793575, 5.2039292296156345, 5.463552712771079, 5.661824779346166, 5.860096845929126, 6.058368956683955, 6.256640988900468, 6.45491305548001, 6.378332782629832, 6.529519171332631, 6.717456542377213, 6.835398162154745, 6.993359168542785, 7.148009338184375, 7.304586577795758, 7.4634849263893175, 7.668071404913257, 7.785674670075932, 7.945396029376635, 8.111619069900609, 8.323904920491882, 8.489436950244789, 8.62104659615015, 8.763899746401965, 8.984982599878846, 9.122693806883749, 9.290110312126899, 9.476223046454201, 9.615850835814562, 9.769591412826784, 9.921879594718726, 10.059116141706546, 10.187746097982288, 10.298550051471265, 10.382078809536544, 10.434000495264597, 10.44448632093743]}, {"Y"=[7.9224735391675205, 7.321473464434564, 6.739168242454245, 6.134745810403829, 5.542921521041388, 4.978309693471735, 4.449970248187061, 3.9578614371636447, 3.5187269716187273, 3.14175802382198, 2.8280843058441714, 2.5937162850227318, 2.4202073591480753, 2.244977169640313, 2.0376215785729492, 1.8310326037758613, 1.6186357963977047, 1.42564842049386, 1.1807351361303358, 0.9756223538774118, 0.7435314685678545, 0.5417446510137208, 0.31677544910316535, 0.1149579734257522, -0.0702125215349173, -0.23172505657020925, -0.37970892354651875, -0.5414576948176312, -0.6468616321179829, -0.7230927377914959, -0.7158640101770734, -0.6262531863681458, -0.45340207002751576, -0.18145982428252616, 0.16153339017341928, 0.5617865094312524, 1.0049769141012719, 1.4863480233133943, 1.9831483476718994, 2.4454162946277305, 2.889593085583598, 3.309204105565798, 3.7288151255446973, 4.148426133001953, 4.568037167454616, 4.987648187434642, 5.483833711602041, 5.960774928198159, 6.431785855959763, 6.923830362042183, 7.402954754910787, 7.88137279475309, 8.378978043446166, 8.875467475222736, 9.352915444903859, 9.838214701876803, 10.336742302958081, 10.831813179411517, 11.320937025460228, 11.8003537185526, 12.287841595036866, 12.801405276612027, 13.293814745353078, 13.788987830920377, 14.289751735273168, 14.760720800003124, 15.252236333764175, 15.74262340416671, 16.245984913005724, 16.733706180572792, 17.228165455837157, 17.73194294963407, 18.24153298822055, 18.751776319543367, 19.26950884612988, 19.79366295038253, 20.326213754641618, 20.87225326020234, 21.42156785783088, 21.97240365912879, 22.479394001104442], "Y"=[-12.295358104289258, -12.368848209891869, -12.366039868118165, -12.299529255201328, -12.152901731107526, -11.930949699264355, -11.63963066634473, -11.278812705532536, -10.855598333720343, -10.382560405732054, -9.868813647407716, -9.361225152127462, -8.904880547516182, -8.467267571883895, -8.005330724036432, -7.549284071982989, -7.0911997781241745, -6.666752009301859, -6.188672905430115, -5.741264902065608, -5.257959416192246, -4.810432906104093, -4.324646840359476, -3.834699942856202, -3.3358684220394967, -2.8429063409679163, -2.357763931437393, -1.8043156929257018, -1.2634138069197096, -0.6582763329381254, -0.026765259453594398, 0.5407122928550108, 1.178982435872069, 1.7392451740487433, 2.240817321179563, 2.6888468030421757, 3.0770269363292453, 3.4127357629657604, 3.6871201234096276, 3.898097856599401, 4.096442391812379, 4.294714458394951, 4.492986524974636, 4.691258585638252, 4.889530667944297, 5.087802734525394, 5.317520478425312, 5.485092092438001, 5.64769889906765, 5.822082651010975, 5.982033823211763, 6.141399821188817, 6.306297137813725, 6.469319852801857, 6.625265800892727, 6.792432009083602, 6.955208301932135, 7.116305233128007, 7.276254787812777, 7.442365859737624, 7.611105388760248, 7.781884247137096, 7.940477658542712, 8.1114206200653, 8.278221745826903, 8.4351654382976, 8.604229739747527, 8.767632595966866, 8.93357746961272, 9.091929680472706, 9.248674993631454, 9.403237050075806, 9.551559622166277, 9.688375317481698, 9.811887463039348, 9.917026770453182, 10.003228584836691, 10.068144755350426, 10.107729465036254, 10.119378871078778, 10.109305075511843]}, {"Y"=[1.3470915265169374, 1.6921924502018477, 2.350947359675299, 2.926007032436896, 3.472919068553876, 4.01553923764964, 4.540771553603303, 5.060339948090165, 5.558610823136398, 6.019770740590945, 6.466417913813986, 6.886028933795981, 7.305639953774969, 7.725250962609034, 8.144861995684934, 8.564473015664918, 9.033292240733939, 9.507748305528745, 9.982559003445736, 10.465812099477526, 10.944605083330368, 11.422232043345485, 11.918421793799222, 12.414200190202452, 12.899637481676528, 13.37678754684273, 13.874783465668319, 14.370744561954087, 14.868407110563963, 15.347734850377055, 15.829260577613933, 16.33800747711995, 16.840800167460728, 17.330629454236842, 17.83149600020578, 18.307170795470793, 18.793936003289474, 19.282694540287146, 19.78369621145204, 20.267635515491328, 20.756809613631752, 21.25179974157784, 21.74713849772317, 22.236508427679524, 22.722656802659756], "Y"=[2.8962835690170365, 3.265562716322244, 3.4006089292605273, 3.512279221773241, 3.5953374904708157, 3.622437769324544, 3.623063809872327, 3.5757747817018526, 3.56036016701454, 3.743209849888086, 4.016917878895559, 4.215189945468877, 4.413462012052612, 4.61173413464184, 4.810006155024352, 5.008278221603526, 4.868806594115014, 5.017139252390996, 5.209509379461617, 5.317736171223016, 5.47536534066575, 5.629232093137066, 5.784437062614739, 5.942659837296325, 6.155411787532055, 6.264698912841051, 6.42392237988264, 6.590981837822474, 6.812082411109792, 6.977514156959353, 7.102822406709091, 7.24110252096422, 7.472616124159055, 7.604691291930131, 7.772210321235591, 7.963262450759516, 8.097906275068672, 8.250045548981548, 8.40009947677207, 8.53394808955574, 8.658191795172698, 8.762449905848245, 8.8369058516278, 8.878040735642243, 8.876062057147013]}, {"Y"=[7.710315740535928, 7.318228037388939, 6.895528781102477, 6.501757566222534, 6.111774833888363, 5.735704462825447, 5.380649609435707, 5.054924570161421, 4.7596024356590885, 4.499092239675365, 4.278166744665951, 4.089102278529083, 3.904755795193055, 3.7046548666886947, 3.495014818056198, 3.282575189342792, 3.0739266292849514, 2.848573410978404, 2.6350002926864415, 2.4176291141079678, 2.2020480421551136, 1.9926645012883535, 1.7956157164989206, 1.6142862728460952, 1.4500919057305408, 1.2986505892402076, 1.1531603649029383, 1.028252179118328, 0.9381582059669654, 0.8768965432058912, 0.8659466285499812, 0.9273761103327463, 0.9961184132684305, 1.1492471661511572, 1.365618593566012, 1.6259734415878775, 1.9305505914189107, 2.2663620157631854, 2.647536860206764, 3.0983319811358476, 3.573148246062948, 3.9927592660414053, 4.412370286021941, 4.8319813185248055, 5.251592327932702, 5.67120334791195, 6.014239863704302, 6.482988467645475, 6.9666646776145456, 7.430488117614067, 7.908617427576298, 8.384677553250869, 8.878122763437181, 9.372550012016466, 9.874318246914124, 10.334836032372968, 10.831836166680331, 11.329470097797818, 11.84476209179978, 12.323889263806183, 12.792812198731816, 13.29241302624446, 13.816067216021146, 14.294624424329601, 14.795696018423165, 15.281249604081424, 15.758046881797691, 16.24360281259667, 16.740135975558726, 17.21729941118971, 17.697701008012572, 18.179599450331803, 18.656792581905684, 19.124588908434816, 19.585808275078925, 20.051376885574644, 20.517546642391945, 20.99031700331575, 21.45747691009842, 21.940618256655217, 22.447608598630868], "Y"=[-10.70948639810373, -10.768851501394227, -10.773698390308322, -10.742191022481514, -10.657439960127398, -10.52156928101113, -10.338156146215423, -10.114144305421542, -9.845534928412233, -9.535421794598271, -9.192602940142088, -8.792172667355606, -8.308126041009189, -7.812026379085751, -7.345024018399936, -6.876213405347107, -6.426272269508127, -5.935120632545394, -5.521505119616947, -5.047999798768626, -4.600137704349835, -4.136020874717464, -3.7138838228732727, -3.2761172269068966, -2.837195735363109, -2.3760547770738345, -1.8991663469164366, -1.4944594171009975, -1.0449827814742285, -0.6524196535491742, -0.2673377084370725, 0.15830412292045987, 0.5015679626686349, 0.8508652409058738, 1.187167083685631, 1.4940639050112943, 1.771916455237049, 2.0157467968022704, 2.231583141944811, 2.437378476871852, 2.6498075579368594, 2.848079624517664, 3.0463516910981228, 3.2446237635961372, 3.442895834068181, 3.6411679006489104, 3.8079942899104933, 3.972712173496366, 4.139751736152054, 4.304420660079245, 4.464039995334728, 4.6226225761415085, 4.786147622632705, 4.948494763708864, 5.1126061835115255, 5.271456251848721, 5.43373465243814, 5.595668001049872, 5.764432278430686, 5.930443066452188, 6.09288119931919, 6.259087021699353, 6.428111182822922, 6.59341810511168, 6.760321754935594, 6.922204842602915, 7.086285179001638, 7.248086732121628, 7.411797351666064, 7.566761628321898, 7.719120690821865, 7.867136904452785, 8.006386664257533, 8.132415557859344, 8.243463199248932, 8.337918310717816, 8.414709864120713, 8.472506653347954, 8.508132472051695, 8.519694624675884, 8.509620829108949]}, {"Y"=[0.8, 0.8, -0.8, -0.8, 0.8], "Y"=[0.0, 3.2, 3.2, 0.0, 0.0]}, {"Y"=[7.816394639851724, 7.319850750911751, 6.817348511778361, 6.318251688313182, 5.827348177464875, 5.357007078148591, 4.915309928811384, 4.506393003662533, 4.139164703638908, 3.8204251317486726, 3.553125525255061, 3.3414092817759076, 3.162481577170565, 2.974816018164504, 2.7663181983145737, 2.5568038965593267, 2.346281212841328, 2.137110915736132, 1.9078677144083886, 1.6966257339926898, 1.4727897553614842, 1.267204576151037, 1.056195582801043, 0.8646221231359237, 0.6899396920978118, 0.5334627663349991, 0.38672572067820976, 0.24339724215034841, 0.1456482869244913, 0.07690190270719764, 0.07504130918645387, 0.15056146198230025, 0.2713581716204574, 0.48389367093431557, 0.7635759918697156, 1.093879975509565, 1.4677637527600913, 1.8763550195382899, 2.3153426039393317, 2.771874137881789, 3.231370665823273, 3.6509816858036017, 4.070592705783319, 4.490203725763379, 4.909814747693659, 5.329425767673296, 5.749036787653171, 6.221881697921817, 6.699225266787154, 7.177159239828125, 7.6557860912435425, 8.133025174001979, 8.628550403441674, 9.124008743619601, 9.613616845908991, 10.086525367124885, 10.584289234819206, 11.080641638604668, 11.582849558630004, 12.062121491179392, 12.540326896884341, 13.046909151428244, 13.554940980687112, 14.041806127624989, 14.542723876848166, 15.020985202042274, 15.505141607780933, 15.99311310838169, 16.493060444282225, 16.97550279588125, 17.462933231924865, 17.955771199982937, 18.449162785063116, 18.938182613989092, 19.427658560604403, 19.922519917978587, 20.42188019851678, 20.931285131759044, 21.43952238396465, 21.956510957892004, 22.463501299867655], "Y"=[-11.502422251196494, -11.568849855643048, -11.569869129213243, -11.520860138841421, -11.405170845617462, -11.226259490137743, -10.988893406280077, -10.696478505477039, -10.350566631066288, -9.958991100165163, -9.530708293774902, -9.076698909741534, -8.606503294262685, -8.139646975484823, -7.675177371218184, -7.212748738665048, -6.758736023816151, -6.300936320923626, -5.855089012523531, -5.394632350417117, -4.92904856027104, -4.473226890410778, -4.019265331616374, -3.5554085848815493, -3.086532078701303, -2.6094805590208754, -2.1284651391769147, -1.6493875550133497, -1.154198294196969, -0.6553479932436498, -0.14705148394533343, 0.3495082078877353, 0.840275199270352, 1.2950552074773085, 1.7139922024325969, 2.091455354026735, 2.424471695783147, 2.7142412798840154, 2.9593516326772193, 3.1677381667356266, 3.373124974874619, 3.571397041456308, 3.76966910803638, 3.9679411746171946, 4.166213251006239, 4.364485317587152, 4.562757384167902, 4.728902132967184, 4.893725317609852, 5.06325165554511, 5.223036909273246, 5.382011198665163, 5.546222380223215, 5.708907308255361, 5.868935992202126, 6.031944130466162, 6.194471477185138, 6.35598661708894, 6.520343533121731, 6.686404463094906, 6.851993294039719, 7.0204856344182245, 7.184294420682817, 7.35241936258849, 7.5192717503812485, 7.678685140450257, 7.845257459374583, 8.007859664044247, 8.172687410639393, 8.329345654397303, 8.483897842226659, 8.635186977264295, 8.778973143211905, 8.910395437670521, 9.02767533114414, 9.127472540585499, 9.208969224478702, 9.27032570434919, 9.307930968543975, 9.319536747877331, 9.309462952310396]}]
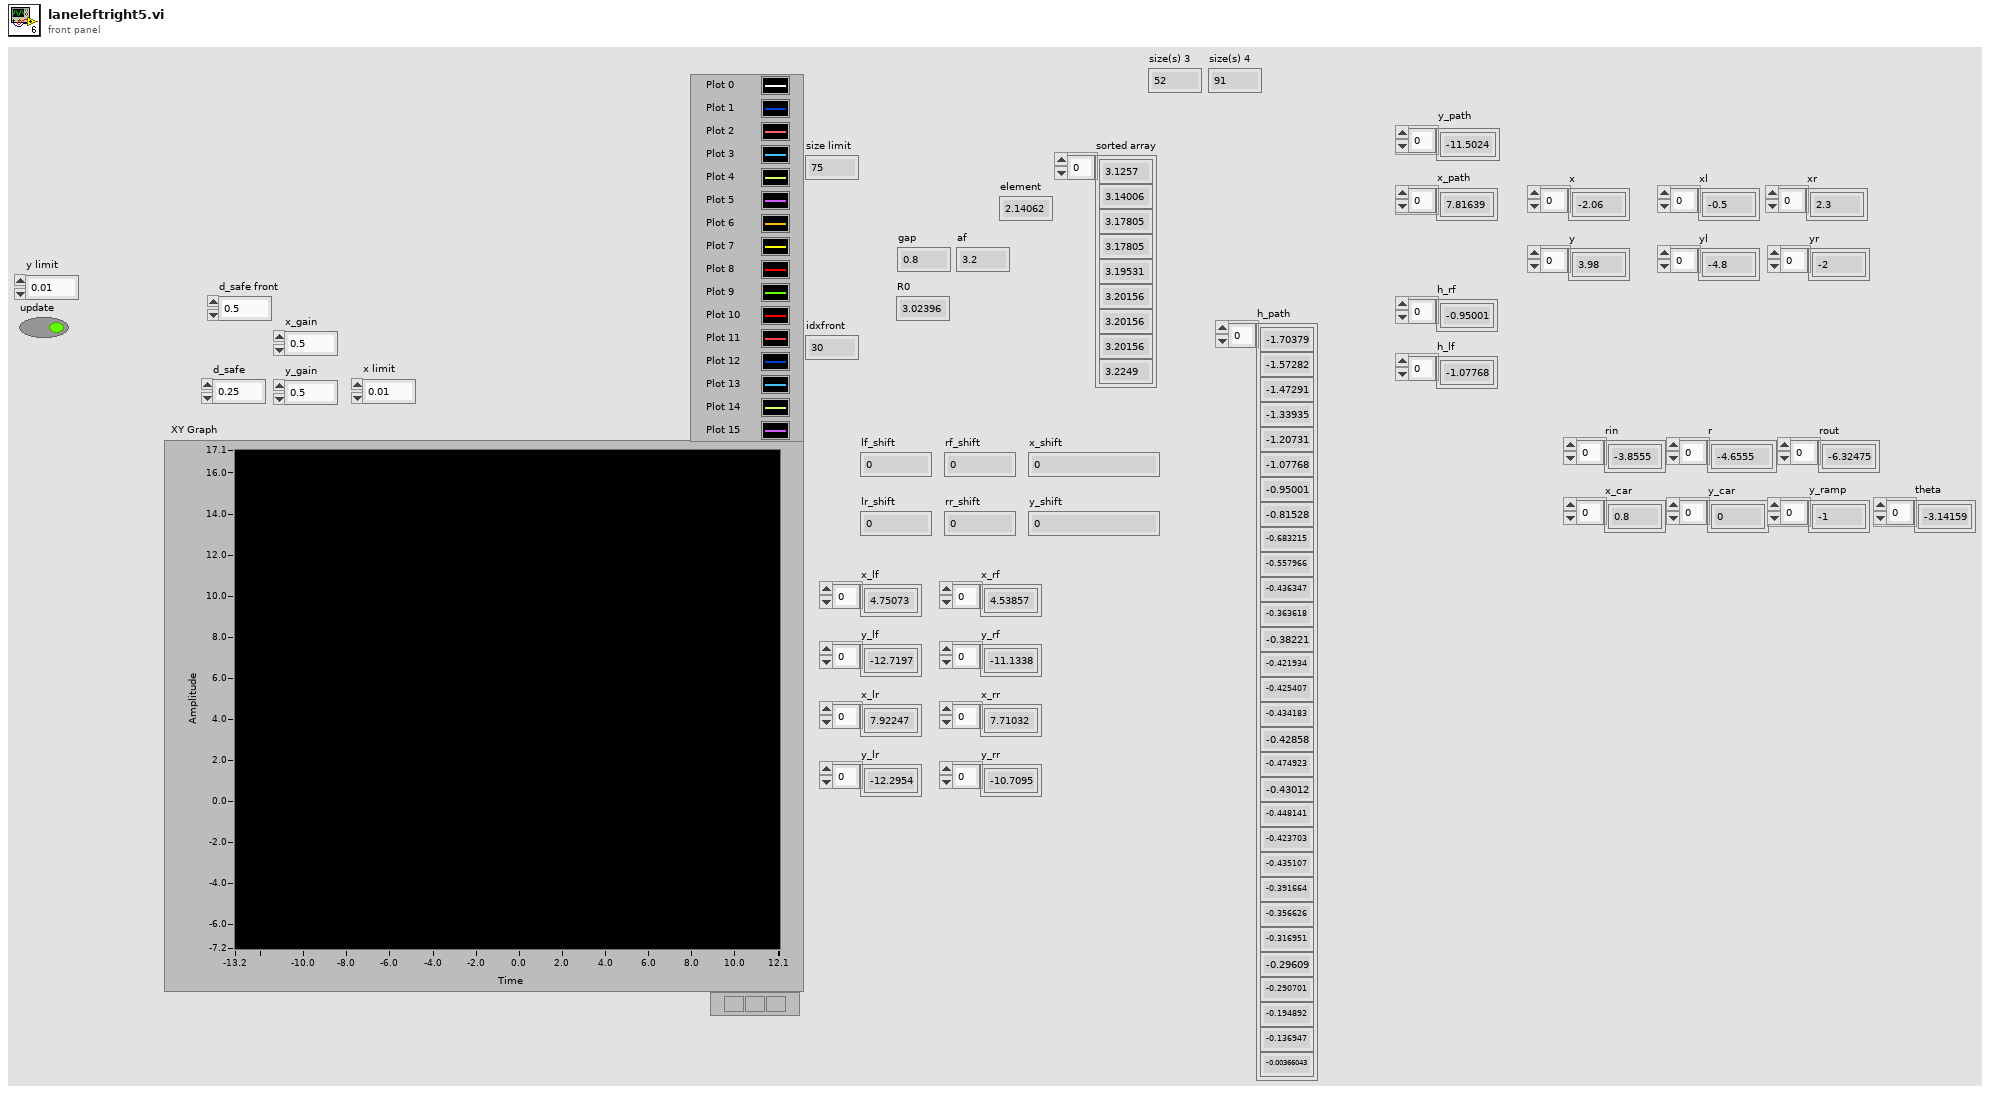
[diagram p1: front panel]
types:
  T1 = cluster{"C_Wheel base":dbl, "ratio_steer":dbl, "Overall width":dbl, "af":dbl, "turn radius":dbl, "eval":dbl, "ap":dbl, "an":dbl, "Vmax":dbl, "mu":dbl, "Vlast":dbl}
  T2 = cluster{"hash":i64, "sys time":i64, "size":i64, "x":dbl[], "y":dbl[], "point_flag":i32[]}
  T3 = cluster{"delta":bool, "Rotational position":dbl, "Rotational position":dbl}[]
  T4 = cluster{"Rotational position":bool, "Numeric":i32, "Rotational position":dbl, "Rotational position":dbl}[]
  T5 = cluster{"Numeric":i32, "Rotational position":dbl, "Rotational position":dbl}[]
  T6 = cluster{bool, "Rotational position":dbl, "Rotational position":dbl}[]
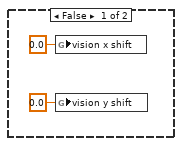
[diagram p2: hidden frame]
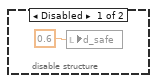
[diagram p4: hidden frame]
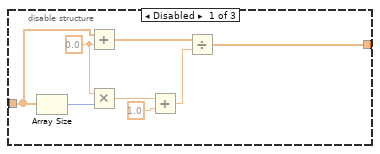
[diagram p5: hidden frame]
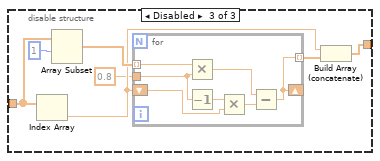
[diagram p6: hidden frame]
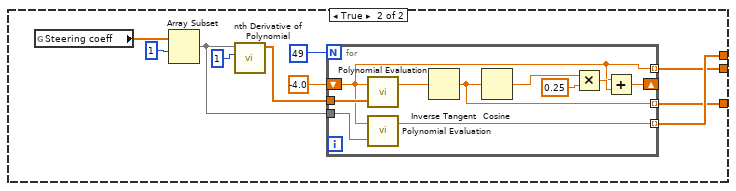
[diagram p8: hidden frame]
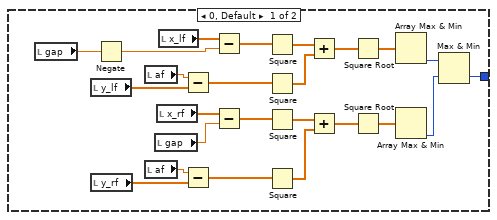
[diagram p9: hidden frame]
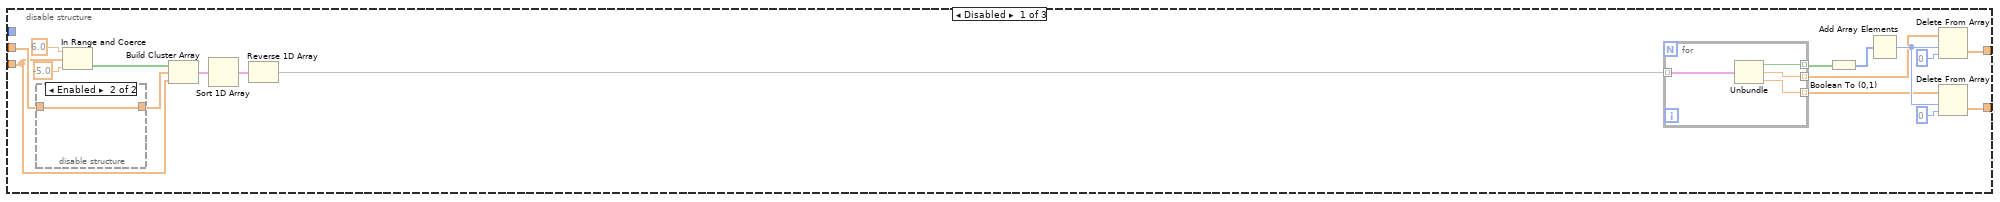
[diagram p10: hidden frame]
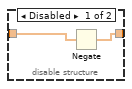
[diagram p11: hidden frame]
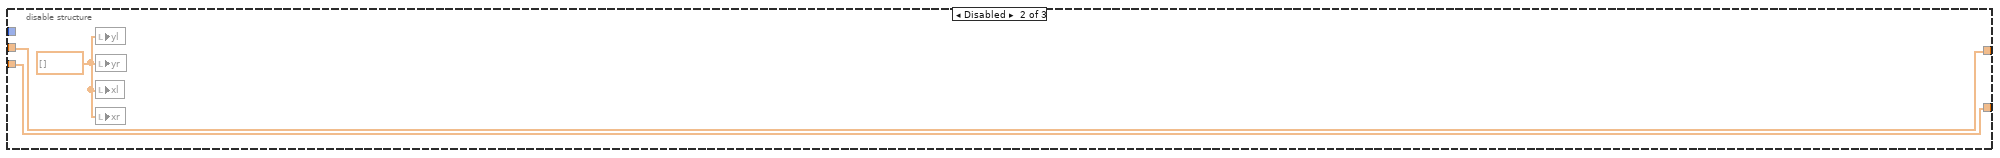
[diagram p12: hidden frame]
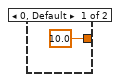
[diagram p13: hidden frame]
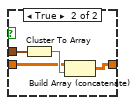
[diagram p15: hidden frame]
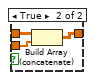
[diagram p19: hidden frame]
diagram:
  n1 = case shown="True" "update" {
    frame False {
      n2 = global write "G_SEN.vi" "vision x shift"(0.0 ("vision x shift")) -> ()
      n3 = global write "G_SEN.vi" "vision y shift"(0.0 ("vision y shift")) -> ()
    }
    frame True {
      n4 = flat-sequence {
        frame #0 {
          n5 = First Call?() -> (First Call?: T/F=w4:bool)
          n6 = case shown="True" w4 {
            frame False {
            }
            frame True {
              n7 = flat-sequence {
                frame #0 {
                  w23 = 3.141592653589793
                  n8 = global read "G_ALL.vi" "CARSPEC"() -> (w41:T1)
                  n9 = Negate(x=w23) -> (-x=w24:dbl)
                  n10 = Unbundle By Name(w41) -> ("C_Wheel base"=w21:dbl, "turn radius"=w40:dbl, "Overall width"=w35:dbl, "C_Wheel base"=w7:dbl)
                  n11 = call-poly <vilib>:"Ramp Pattern.vi"("start"=w24, "end"=w23, "delta"=0.01) -> ("Ramp Pattern"=w18:dbl[])  [unwired: 6 in, 2 out]
                  n12 = Divide(x=w21, y=w40) -> (x/y=w39:dbl)
                  n13 = Multiply(x=w35, y=0.5) -> (x*y=w20:dbl)
                  n14 = Add(x=w7, y=0.5) -> (x+y=w5:dbl)
                  "af" <- w5
                  n15 = Inverse Tangent(1:w39) -> (0:w38:dbl)
                  n16 = Negate(x=3.141592653589793) -> (-x=w15:dbl)
                  n17 = Add(x=w20, y=0.1) -> (x+y=w10:dbl)
                  n18 = Negate(x=w38) -> (-x=w11:dbl)
                  n19 = Build Array (concatenate)(w18, w15) -> (→"theta":dbl[])
                  n20 = Max & Min(x=w10, y=0.8) -> (min(x,y)=w9:dbl)  [unwired: 1 out]
                  "gap" <- w9
                  n21 = call-poly <vilib>:"Ramp Pattern.vi"("start"=w11, "end"=w38, "delta"=0.025) -> ("Ramp Pattern"=w36:dbl[])  [unwired: 6 in, 2 out]
                  n22 = Square(x=w5) -> (x^2=w29:dbl)
                  n23 = Tangent(1:w36) -> (0:w33:dbl[])
                  n24 = Divide(x=w21, y=w33) -> (x/y=w14:dbl[])
                  "r" <- w14
                  n25 = Sign(1:w33) -> (0:w32:dbl[])
                  n26 = Multiply(x=w32, y=w9) -> (x*y=w31:dbl[])
                  n27 = Subtract(x=w14, y=w31) -> (x-y=→"rin":dbl[])
                  n28 = Add(x=w14, y=w31) -> (x+y=w27:dbl[])
                  n29 = Square(x=w27) -> (x^2=w30:dbl[])
                  n30 = Sign(1:w27) -> (0:w25:dbl[])
                  n31 = Add(x=w30, y=w29) -> (x+y=w28:dbl[])
                  n32 = Square Root(x=w28) -> (sqrt(x)=w26:dbl[])
                  n33 = Multiply(x=w25, y=w26) -> (x*y=→"rout":dbl[])
                }
                frame #1 {
                  w47 = 0.0 ("element")
                  n34 = disable-structure shown="Enabled" {
                    frame Disabled {
                      n35 = local write "d_safe"(0.6 ("d_safe")) -> ()
                    }
                    frame Enabled {
                    }
                  }
                  n36 = local read "gap"() -> (w54:dbl)
                  n37 = local read "af"() -> (w49:dbl)
                  n38 = Negate(x=w54) -> (-x=w52:dbl)
                  n39 = Build Array(0.0 ("element"), w49, w49, w47, w47) -> (→"y_car":dbl[])
                  n40 = local read "gap"() -> (w53:dbl)
                  n41 = local read "gap"() -> (w51:dbl)
                  n42 = call-poly <vilib>:"Ramp Pattern.vi"("start"=-1.0, "end"=6.0, "delta"=0.25) -> ("Ramp Pattern"=→"y_ramp":dbl[])  [unwired: 6 in, 2 out]
                  n43 = Build Array(w53, w53, w52, w52, w51) -> (→"x_car":dbl[])
                }
              }
            }
          }
        }
        frame #1 {
          n44 = disable-structure shown="Enabled" {
            disable-tunnel: [w94 _] -> w58
            frame Enabled {
              n45 = global read "G_ALL.vi" "dist"() -> (w101:dbl[])
              n46 = global read "G_ALL.vi" "mission num"() -> (w96:i32)
              n47 = Threshold 1D Array(2:-4.0 ("threshold y"), 3:w101) -> (0:w99:dbl)  [unwired: 1 in]
              n48 = Round Toward -Infinity(1:w99) -> (0:w98:dbl)
              n49 = To Long Integer(number=w98) -> (32bit integer=w93:i32)
              n50 = Equal?(x=w96, y=6) -> (x = y?=w95:bool)
              n51 = Select(t=0, s=w95, f=w93) -> (s? t:f=w94:i32)
            }
            frame Disabled {
            }
          }
          n52 = global read "G_ALL.vi" "Steering coeff"() -> (w66:dbl[])
          n53 = Index Array(array=w66, index=0) -> (element=→"R0":dbl)
          n54 = global read "G_ALL.vi" "map_track 2"() -> (w60:dbl[][])
          n55 = global read "G_ALL.vi" "v origin 2"() -> (w62:dbl[])
          n56 = Array Subset(array=w60, index (row)=w58) -> (w59:dbl[][])  [unwired: 3 in]
          n57 = Empty Array?(array=w59) -> (empty?=w63:bool)
          n58 = Array Subset(array=w62, index=w58) -> (w61:dbl[])  [unwired: 1 in]
          n59 = case shown="False" w63 {
            tunnel: [w134 w153] -> w68
            tunnel: [w132 w144] -> w57
            tunnel: [w133 w152] -> w67
            tunnel: w59 -> [w131 _]
            tunnel: w61 -> [w102 _]
            frame False {
              n60 = Array Size(array=w131) -> (size(s)=w128:i32[])
              n61 = Index Array(array=w102, index=0) -> (element=w109:dbl)
              "element" <- w109
              n62 = Index Array(array=w128, index=0) -> (element=w126:i32)
              n63 = Less Than 0?(x=w109) -> (x < 0?=w107:bool)
              n64 = Decrement(x=w126) -> (x-1=w118:i32)
              n65 = Array Subset(array=w131, index (row)=1 ("index")) -> (w124:dbl[][])  [unwired: 3 in]
              n66 = Decrement(x=w118) -> (x-1=w117:i32)
              n67 = Array Subset(array=w131, index (row)=0 ("index"), length (row)=w118) -> (w125:dbl[][])  [unwired: 2 in]
              n68 = Subtract(x=w124, y=w125) -> (x-y=w123:dbl[][])
              n69 = Select(t=3.141592653589793, s=w107, f=0.0) -> (s? t:f=w105:dbl)
              n70 = Index Array(array=w123, index (col) #1=0 ("disabled index (col)"), index (col) #2=1 ("index (col)")) -> (element #1=w120:dbl[], element #2=w119:dbl[])  [unwired: 2 in]
              n71 = Inverse Tangent (2 Input)(1:w119, 2:w120) -> (0:w115:dbl[])
              n72 = Index Array(array=w115, index=w117) -> (element=w111:dbl)
              n73 = Delete From Array(array=w115, index=0) -> (deleted portion=w108:dbl, array with subset deleted=w113:dbl[])  [unwired: 1 in]
              n74 = call "headingoperater.vi"("h1"=w105, "h2"=w108) -> ("h2-h1"=w104:dbl)  [unwired: 8 in, 1 out]
              n75 = for {
                tunnel: w113 -> [w137] mode=indexing
                shift-right: [w138] -> _
                shift-left: w104 -> [w136]
                tunnel: [w138] -> w112 mode=indexing
                n76 = call "headingoperater.vi"("h1"=w136, "h2"=w137) -> ("h2-h1"=w135:dbl)  [unwired: 8 in, 1 out]
                n77 = call "headingoperater.vi"("h1"=3.141592653589793, "h2"=w137) -> ("h2-h1"=w140:dbl)  [unwired: 8 in, 1 out]
                n78 = Absolute Value(x=w135) -> (abs(x)=w143:dbl)
                n79 = Less?(x=w143, y=1.5707963267948966) -> (x < y?=w141:bool)
                n80 = Select(t=w137, s=w141, f=w140) -> (s? t:f=w138:dbl)
              }
              n81 = Build Array (concatenate)(w104, w112, w111) -> (w132:dbl[])
              n82 = Index Array(array=w131, index (col) #1=0 ("disabled index (col)")) -> (element #1=w134:dbl[], element #2=w133:dbl[])  [unwired: 3 in]
            }
            frame True {
              n83 = global read "G_ALL.vi" "Steering coeff"() -> (w145:dbl[])
              n84 = Array Subset(array=w145, index=1) -> (w147:dbl[])  [unwired: 1 in]
              n85 = call-poly <vilib>:"nth Derivative of Polynomial.vi"("order"=1, "P(x)"=w147) -> ("Nth Derivative of P(x)"=w148:dbl[])  [unwired: 8 in, 1 out]
              n86 = for {
                N: 49 -> [_]
                shift-right: [w154] -> _
                shift-left: -4.0 -> [w155]
                tunnel: w148 -> [w163]
                tunnel: w147 -> [w159]
                tunnel: [w158] -> w153 mode=indexing
                tunnel: [w155] -> w152 mode=indexing
                tunnel: [w157] -> w144 mode=indexing
                n87 = call-poly <vilib>:"Polynomial Evaluation.vi"("P(x)"=w163, "a"=w155) -> ("P(a)"=w162:dbl)  [unwired: 1 out]
                n88 = call-poly <vilib>:"Polynomial Evaluation.vi"("P(x)"=w159, "a"=w155) -> ("P(a)"=w158:dbl)  [unwired: 1 out]
                n89 = Inverse Tangent(1:w162) -> (0:w157:dbl)
                n90 = Cosine(x=w157) -> (cos(x)=w161:dbl)
                n91 = Multiply(x=w161, y=0.25) -> (x*y=w156:dbl)
                n92 = Add(x=w155, y=w156) -> (x+y=w154:dbl)
              }
            }
          }
          "y_path" <- w67
          "x_path" <- w68
          n93 = disable-structure shown="Enabled" {
            disable-tunnel: w57 -> [w70 w77 w79]
            disable-tunnel: [w69 w77 w80] -> w56
            frame Disabled {
              w73 = 0.0
              n94 = Array Size(array=w70) -> (size(s)=w72:i32)
              n95 = Add(x=w70, y=w73) -> (x+y=w71:dbl[])
              n96 = Multiply(x=w73, y=w72) -> (x*y=w74:dbl)
              n97 = Add(x=w74, y=1.0) -> (x+y=w76:dbl)
              n98 = Divide(x=w71, y=w76) -> (x/y=w69:dbl[])
            }
            frame Enabled {
            }
            frame Disabled {
              n99 = Index Array(array=w79) -> (element=w81:dbl)  [unwired: 1 in]
              n100 = Array Subset(array=w79, index=1) -> (w83:dbl[])  [unwired: 1 in]
              n101 = for {
                tunnel: w83 -> [w91] mode=indexing
                tunnel: 0.8 ("LPFGAIN") -> [w90]
                shift-right: [w85] -> _
                shift-left: w81 -> [w86]
                tunnel: [w85] -> w82 mode=indexing
                n102 = Multiply(x=w91, y=w90) -> (x*y=w88:dbl)
                n103 = Decrement(x=w90) -> (x-1=w89:dbl)
                n104 = Multiply(x=w89, y=w86) -> (x*y=w87:dbl)
                n105 = Subtract(x=w88, y=w87) -> (x-y=w85:dbl)
              }
              n106 = Build Array (concatenate)(w81, w82) -> (w80:dbl[])
            }
          }
          "h_path" <- w56
        }
        frame #2 {
          n107 = local read "y_path"() -> (w168:dbl[])
          n108 = local read "h_path"() -> (w169:dbl[])
          n109 = local read "x_path"() -> (w167:dbl[])
          n110 = local read "gap"() -> (w179:dbl)
          n111 = local read "gap"() -> (w164:dbl)
          n112 = local read "af"() -> (w165:dbl)
          n113 = Negate(x=w179) -> (-x=w178:dbl)
          n114 = for {
            tunnel: w167 -> [w190] mode=indexing
            tunnel: w168 -> [w189] mode=indexing
            tunnel: w169 -> [w191] mode=indexing
            tunnel: [w194] -> w170 mode=indexing
            tunnel: [w193] -> w171 mode=indexing
            tunnel: [w187] -> w172 mode=indexing
            tunnel: [w186] -> w173 mode=indexing
            tunnel: w165 -> [w184]
            tunnel: w164 -> [w183]
            n115 = call "rotm_siso.vi"("angle[rad]"=w191, "reverse"=TRUE, "y0"=w190, "x0"=w189, "y"=w183, "x"=0.0) -> ("y'"=w186:dbl, "x'"=w187:dbl)  [unwired: 4 in]
            n116 = call "rotm_siso.vi"("angle[rad]"=w191, "reverse"=TRUE, "y0"=w190, "x0"=w189, "y"=w183, "x"=w184) -> ("y'"=w193:dbl, "x'"=w194:dbl)  [unwired: 4 in]
          }
          "x_rf" <- w171
          "y_rf" <- w170
          "y_rr" <- w172
          "x_rr" <- w173
          n117 = local read "y_path"() -> (w181:dbl[])
          n118 = local read "h_path"() -> (w180:dbl[])
          n119 = local read "x_path"() -> (w182:dbl[])
          n120 = local read "af"() -> (w166:dbl)
          n121 = for {
            tunnel: w182 -> [w202] mode=indexing
            tunnel: w181 -> [w201] mode=indexing
            tunnel: w180 -> [w203] mode=indexing
            tunnel: [w206] -> w177 mode=indexing
            tunnel: [w205] -> w176 mode=indexing
            tunnel: w178 -> [w200]
            tunnel: [w198] -> w175 mode=indexing
            tunnel: [w197] -> w174 mode=indexing
            tunnel: w166 -> [w195]
            n122 = call "rotm_siso.vi"("angle[rad]"=w203, "reverse"=TRUE, "y0"=w202, "x0"=w201, "y"=w200, "x"=0.0) -> ("y'"=w197:dbl, "x'"=w198:dbl)  [unwired: 4 in]
            n123 = call "rotm_siso.vi"("angle[rad]"=w203, "reverse"=TRUE, "y0"=w202, "x0"=w201, "y"=w200, "x"=w195) -> ("y'"=w205:dbl, "x'"=w206:dbl)  [unwired: 4 in]
          }
          "x_lf" <- w176
          "y_lf" <- w177
          "y_lr" <- w175
          "x_lr" <- w174
        }
        frame #3 {
          n124 = global read "G_ALL.vi" "mission num"() -> (w207:i32)
          n125 = local read "y_path"() -> (w246:dbl[])
          n126 = local read "y_rf"() -> (w210:dbl[])
          n127 = local read "x_lf"() -> (w214:dbl[])
          n128 = local read "y_lf"() -> (w213:dbl[])
          n129 = local read "x_rf"() -> (w209:dbl[])
          n130 = case shown="60" w207 {
            tunnel: [w250 _] -> w208
            frame 0, Default {
              n131 = local read "gap"() -> (w267:dbl)
              n132 = local read "y_lf"() -> (w269:dbl[])
              n133 = local read "y_rf"() -> (w270:dbl[])
              n134 = Negate(x=w267) -> (-x=w266:dbl)
              n135 = local read "af"() -> (w265:dbl)
              n136 = local read "af"() -> (w251:dbl)
              n137 = local read "gap"() -> (w252:dbl)
              n138 = local read "x_rf"() -> (w271:dbl[])
              n139 = local read "x_lf"() -> (w268:dbl[])
              n140 = Subtract(x=w265, y=w269) -> (x-y=w255:dbl[])
              n141 = Subtract(x=w251, y=w270) -> (x-y=w253:dbl[])
              n142 = Subtract(x=w268, y=w266) -> (x-y=w256:dbl[])
              n143 = Subtract(x=w271, y=w252) -> (x-y=w254:dbl[])
              n144 = Square(x=w256) -> (x^2=w257:dbl[])
              n145 = Square(x=w255) -> (x^2=w258:dbl[])
              n146 = Square(x=w254) -> (x^2=w264:dbl[])
              n147 = Square(x=w253) -> (x^2=w263:dbl[])
              n148 = Add(x=w257, y=w258) -> (x+y=w259:dbl[])
              n149 = Add(x=w264, y=w263) -> (x+y=w262:dbl[])
              n150 = Square Root(x=w259) -> (sqrt(x)=w260:dbl[])
              n151 = Square Root(x=w262) -> (sqrt(x)=w261:dbl[])
              n152 = Array Max & Min(array=w260) -> (min index (indices)=w249:i32)  [unwired: 3 out]
              n153 = Array Max & Min(array=w261) -> (min index (indices)=w248:i32)  [unwired: 3 out]
              n154 = Max & Min(x=w249, y=w248) -> (min(x,y)=w250:i32)  [unwired: 1 out]
            }
            frame 60 {
            }
          }
          "idxfront" <- w208
          n155 = for {
            tunnel: w214 -> [w296] mode=indexing
            tunnel: w213 -> [w295] mode=indexing
            tunnel: [w285] -> w212 mode=indexing
            n156 = local read "x_path"() -> (w297:dbl[])
            n157 = local read "y_path"() -> (w294:dbl[])
            n158 = Subtract(x=w297, y=w296) -> (x-y=w289:dbl[])
            n159 = Subtract(x=w295, y=w294) -> (x-y=w288:dbl[])
            n160 = Square(x=w289) -> (x^2=w290:dbl[])
            n161 = Square(x=w288) -> (x^2=w291:dbl[])
            n162 = Add(x=w290, y=w291) -> (x+y=w292:dbl[])
            n163 = Square Root(x=w292) -> (sqrt(x)=w293:dbl[])
            n164 = local read "h_path"() -> (w287:dbl[])
            n165 = Array Max & Min(array=w293) -> (min index (indices)=w286:i32)  [unwired: 3 out]
            n166 = Index Array(array=w287, index=w286) -> (element=w285:dbl)
          }
          "h_lf" <- w212
          n167 = for {
            tunnel: w209 -> [w283] mode=indexing
            tunnel: w210 -> [w282] mode=indexing
            tunnel: [w272] -> w211 mode=indexing
            n168 = local read "x_path"() -> (w284:dbl[])
            n169 = local read "y_path"() -> (w281:dbl[])
            n170 = Subtract(x=w284, y=w283) -> (x-y=w276:dbl[])
            n171 = Subtract(x=w282, y=w281) -> (x-y=w275:dbl[])
            n172 = Square(x=w276) -> (x^2=w277:dbl[])
            n173 = Square(x=w275) -> (x^2=w278:dbl[])
            n174 = Add(x=w277, y=w278) -> (x+y=w279:dbl[])
            n175 = Square Root(x=w279) -> (sqrt(x)=w280:dbl[])
            n176 = local read "h_path"() -> (w274:dbl[])
            n177 = Array Max & Min(array=w280) -> (min index (indices)=w273:i32)  [unwired: 3 out]
            n178 = Index Array(array=w274, index=w273) -> (element=w272:dbl)
          }
          "h_rf" <- w211
          n179 = local read "x_path"() -> (w247:dbl[])
          n180 = Array Size(array=w246) -> (size(s)=w244:i32)
          n181 = Build Array(w247, w246) -> (w245:dbl[][])
          n182 = Decrement(x=w244) -> (x-1=w243:i32)
          n183 = Index Array(array=w245, index (col)=w243) -> (element=w218:dbl[])  [unwired: 1 in]
          n184 = Index Array(array=w218, index #1=0 ("index")) -> (element #1=w241:dbl, element #2=w239:dbl)  [unwired: 1 in]
          n185 = Index Array(array=w218, index #1=0 ("index")) -> (element #1=w220:dbl, element #2=w222:dbl)  [unwired: 1 in]
          n186 = local read "y_lf"() -> (w238:dbl[])
          n187 = local read "x_rf"() -> (w221:dbl[])
          n188 = local read "y_rf"() -> (w223:dbl[])
          n189 = local read "x_lf"() -> (w240:dbl[])
          n190 = Subtract(x=w240, y=w241) -> (x-y=w236:dbl[])
          n191 = Subtract(x=w239, y=w238) -> (x-y=w237:dbl[])
          n192 = Subtract(x=w221, y=w220) -> (x-y=w225:dbl[])
          n193 = Subtract(x=w222, y=w223) -> (x-y=w224:dbl[])
          n194 = Square(x=w236) -> (x^2=w235:dbl[])
          n195 = Square(x=w237) -> (x^2=w234:dbl[])
          n196 = Square(x=w225) -> (x^2=w226:dbl[])
          n197 = Square(x=w224) -> (x^2=w227:dbl[])
          n198 = Add(x=w235, y=w234) -> (x+y=w233:dbl[])
          n199 = Add(x=w226, y=w227) -> (x+y=w228:dbl[])
          n200 = Square Root(x=w233) -> (sqrt(x)=w232:dbl[])
          n201 = Square Root(x=w228) -> (sqrt(x)=w229:dbl[])
          n202 = Array Max & Min(array=w232) -> (min index (indices)=w231:i32)  [unwired: 3 out]
          n203 = Array Max & Min(array=w229) -> (min index (indices)=w230:i32)  [unwired: 3 out]
          n204 = Increment(x=w231) -> (x+1=w217:i32)
          n205 = Increment(x=w230) -> (x+1=w216:i32)
          n206 = Max & Min(x=w217, y=w216) -> (max(x,y)=→"size limit":i32)  [unwired: 1 out]
        }
        frame #4 {
          n207 = global read "G_LCM.vi" "VISION_LANE_PT"() -> (w303:T2)
          n208 = Unbundle By Name(w303) -> ("point_flag"=w298:i32[], "x"=w302:dbl[], "y"=w301:dbl[])
          n209 = disable-structure shown="Enabled" {
            disable-tunnel: w302 -> [w320 w331 w347]
            disable-tunnel: [w318 w330 w345] -> w299
            disable-tunnel: [w317 w331 w347] -> w300
            disable-tunnel: w301 -> [w314 w330 w345]
            disable-tunnel: w298 -> [_ _ w346]
            frame Disabled {
              n210 = disable-structure shown="Enabled" {
                disable-tunnel: w320 -> [w323 w324]
                disable-tunnel: [w322 w324] -> w321
                frame Disabled {
                  n211 = Negate(x=w323) -> (-x=w322:dbl[])
                }
                frame Enabled {
                }
              }
              n212 = In Range and Coerce(upper limit=6.0 ("delta"), x=w314, lower limit=-5.0) -> (In Range?=w312:bool[])  [unwired: 1 out]
              n213 = Build Cluster Array(w312, w321, w314) -> (w310:T3)
              n214 = Sort 1D Array(array=w310) -> (sorted array=w311:T3)
              n215 = Reverse 1D Array(array=w311) -> (reversed array=w307:T3)
              n216 = for {
                tunnel: w307 -> [w328] mode=indexing
                tunnel: [w327] -> w305 mode=indexing
                tunnel: [w326] -> w304 mode=indexing
                tunnel: [w325] -> w315 mode=indexing
                n217 = Unbundle(w328) -> ("delta"=w325:bool, "Rotational position"=w327:dbl, "Rotational position"=w326:dbl)
              }
              n218 = Boolean To (0,1)(Boolean=w315) -> (0, 1=w308:i16[])
              n219 = Add Array Elements(numeric array=w308) -> (sum=w316:i16)
              n220 = Delete From Array(array=w305, length=w316, index=0) -> (deleted portion=w317:dbl[])  [unwired: 1 out]
              n221 = Delete From Array(array=w304, length=w316, index=0) -> (deleted portion=w318:dbl[])  [unwired: 1 out]
            }
            frame Disabled {
              w329 = dbl[] [] ("yl")
              n222 = local write "yl"(w329) -> ()
              n223 = local write "yr"(w329) -> ()
              n224 = local write "xl"(w329) -> ()
              n225 = local write "xr"(w329) -> ()
            }
            frame Enabled {
              n226 = global read "G_ALL.vi" "mission num"() -> (w333:i32)
              n227 = case shown="2, 4, 6" w333 {
                tunnel: [10.0 10.0] -> w332
                frame 0, Default {
                }
                frame 2, 4, 6 {
                }
              }
              n228 = In Range and Coerce(upper limit=w332, x=w345, lower limit=-6.0) -> (In Range?=w337:bool[])  [unwired: 1 out]
              n229 = Boolean To (0,1)(Boolean=w337) -> (0, 1=w336:i16[])
              n230 = Build Cluster Array(w337, w346, w347, w345) -> (w343:T4)
              n231 = To Long Integer(number=w336) -> (32bit integer=w335:i32[])
              n232 = Sort 1D Array(array=w343) -> (sorted array=w342:T4)
              n233 = Add Array Elements(numeric array=w335) -> (sum=w334:i32)
              n234 = Reverse 1D Array(array=w342) -> (reversed array=w341:T4)
              n235 = for {
                N: w334 -> [_]
                tunnel: w341 -> [w447] mode=indexing
                tunnel: [w446] -> w340 mode=indexing
                tunnel: [w445] -> w339 mode=indexing
                tunnel: [w444] -> w338 mode=indexing
                n236 = Unbundle(w447) -> ("Numeric"=w446:i32, "Rotational position"=w445:dbl, "Rotational position"=w444:dbl)  [unwired: 1 out]
              }
              n237 = Build Cluster Array(w340, w339, w338) -> (w379:T5)
              n238 = Sort 1D Array(array=w379) -> (sorted array=w378:T5)
              n239 = for {
                tunnel: w378 -> [w451] mode=indexing
                tunnel: [w450] -> w377 mode=indexing
                tunnel: [w448] -> w376 mode=indexing
                tunnel: [w449] -> w366 mode=indexing
                n240 = Unbundle(w451) -> ("Numeric"=w449:i32, "Rotational position"=w450:dbl, "Rotational position"=w448:dbl)
              }
              n241 = Build Array(w377, w376) -> (w375:dbl[][])
              n242 = Not Equal?(x=w366, y=1) -> (x != y?=w364:bool[])
              n243 = Equal?(x=w366, y=-1) -> (x = y?=w370:bool[])
              n244 = Boolean To (0,1)(Boolean=w370) -> (0, 1=w369:i16[])
              n245 = Boolean To (0,1)(Boolean=w364) -> (0, 1=w363:i16[])
              n246 = To Long Integer(number=w369) -> (32bit integer=w368:i32[])
              n247 = To Long Integer(number=w363) -> (32bit integer=w362:i32[])
              n248 = Add Array Elements(numeric array=w368) -> (sum=w367:i32)
              n249 = Add Array Elements(numeric array=w362) -> (sum=w360:i32)
              n250 = Transpose 2D Array(2D array=w375) -> (transposed array=w361:dbl[][])
              n251 = Array Subset(array=w361, index (row)=w360) -> (w358:dbl[][])  [unwired: 3 in]
              n252 = Array Subset(array=w361, index (row)=0 ("index"), length (row)=w367) -> (w373:dbl[][])  [unwired: 2 in]
              n253 = Index Array(array=w373, index (col) #1=0 ("disabled index (col)")) -> (element #1=w352:dbl[], element #2=w350:dbl[])  [unwired: 3 in]
              n254 = Index Array(array=w358, index (col) #1=0 ("disabled index (col)")) -> (element #1=w357:dbl[], element #2=w355:dbl[])  [unwired: 3 in]
              n255 = disable-structure shown="Enabled" {
                disable-tunnel: w357 -> [w415 w441]
                disable-tunnel: [w414 w441] -> w356
                disable-tunnel: w355 -> [w413 w440]
                disable-tunnel: [w412 w440] -> w353
                disable-tunnel: w352 -> [w411 w443]
                disable-tunnel: [w410 w443] -> w351
                disable-tunnel: w350 -> [w409 w442]
                disable-tunnel: [w408 w442] -> w348
                frame Enabled {
                  w394 = 10.0
                  w407 = 10.0
                  n256 = Multiply(x=w411, y=w407) -> (x*y=w406:dbl[])
                  n257 = Multiply(x=w407, y=w409) -> (x*y=w405:dbl[])
                  n258 = Multiply(x=w415, y=w394) -> (x*y=w393:dbl[])
                  n259 = Multiply(x=w394, y=w413) -> (x*y=w392:dbl[])
                  n260 = Round To Nearest(number=w406) -> (nearest integer value=w403:dbl[])
                  n261 = Round To Nearest(number=w405) -> (nearest integer value=w404:dbl[])
                  n262 = Round To Nearest(number=w393) -> (nearest integer value=w390:dbl[])
                  n263 = Round To Nearest(number=w392) -> (nearest integer value=w391:dbl[])
                  n264 = Build Cluster Array(w403, w404) -> (w402:cluster{dbl, dbl}[])
                  n265 = Build Cluster Array(w390, w391) -> (w389:cluster{dbl, dbl}[])
                  n266 = Sort 1D Array(array=w402) -> (sorted array=w401:cluster{dbl, dbl}[])
                  n267 = Sort 1D Array(array=w389) -> (sorted array=w388:cluster{dbl, dbl}[])
                  n268 = for {
                    tunnel: w401 -> [w416] mode=indexing
                    shift-right: [w416] -> _
                    shift-left: cluster{dbl, dbl} {inf, inf} ("output cluster") -> [w422]
                    shift-right: [w418] -> w398
                    shift-left: dbl[][] [] -> [w417]
                    n269 = Not Equal?(x=w422, y=w416) -> (x != y?=w421:cluster{bool, bool})
                    n270 = Cluster To Array(cluster=w421) -> (array=w420:bool[])
                    n271 = Or Array Elements(Boolean array=w420) -> (logical OR=w419:bool)
                    n272 = case shown="True" w419 {
                      tunnel: w416 -> [_ w427]
                      tunnel: [w423 w425] -> w418
                      tunnel: w417 -> [w423 w424]
                      frame False {
                      }
                      frame True {
                        n273 = Cluster To Array(cluster=w427) -> (array=w426:dbl[])
                        n274 = Build Array (concatenate)(w424, w426) -> (w425:dbl[][])
                      }
                    }
                  }
                  n275 = for {
                    tunnel: w388 -> [w428] mode=indexing
                    shift-right: [w428] -> _
                    shift-left: cluster{dbl, dbl} {inf, inf} ("output cluster") -> [w434]
                    shift-right: [w430] -> w385
                    shift-left: dbl[][] [] -> [w429]
                    n276 = Not Equal?(x=w434, y=w428) -> (x != y?=w433:cluster{bool, bool})
                    n277 = Cluster To Array(cluster=w433) -> (array=w432:bool[])
                    n278 = Or Array Elements(Boolean array=w432) -> (logical OR=w431:bool)
                    n279 = case shown="False" w431 {
                      tunnel: w428 -> [_ w439]
                      tunnel: [w435 w437] -> w430
                      tunnel: w429 -> [w435 w436]
                      frame False {
                      }
                      frame True {
                        n280 = Cluster To Array(cluster=w439) -> (array=w438:dbl[])
                        n281 = Build Array (concatenate)(w436, w438) -> (w437:dbl[][])
                      }
                    }
                  }
                  n282 = Multiply(x=w398, y=0.1) -> (x*y=w396:dbl[][])
                  n283 = Multiply(x=w385, y=0.1) -> (x*y=w383:dbl[][])
                  n284 = Index Array(array=w396, index (col) #1=0 ("disabled index (col)")) -> (element #1=w410:dbl[], element #2=w408:dbl[])  [unwired: 3 in]
                  n285 = Index Array(array=w383, index (col) #1=0 ("disabled index (col)")) -> (element #1=w414:dbl[], element #2=w412:dbl[])  [unwired: 3 in]
                }
                frame Disabled {
                }
              }
              "xl" <- w351
              "yl" <- w348
              "xr" <- w356
              "yr" <- w353
              n286 = Array Size(array=w348) -> (size(s)=→"size(s) 4":i32)
              n287 = Array Size(array=w353) -> (size(s)=→"size(s) 3":i32)
            }
          }
          "x" <- w300
          "y" <- w299
        }
        frame #5 {
          n288 = disable-structure shown="Enabled" {
            frame Enabled {
              n289 = flat-sequence {
                frame #0 {
                  n290 = local read "xl"() -> (w453:dbl[])
                  n291 = Empty Array?(array=w453) -> (empty?=w452:bool)
                  n292 = case shown="False" w452 {
                    frame False {
                      n293 = local read "xr"() -> (w468:dbl[])
                      n294 = local read "yr"() -> (w467:dbl[])
                      n295 = for {
                        tunnel: w468 -> [w481] mode=indexing
                        tunnel: w467 -> [w479] mode=indexing
                        tunnel: [w472] -> w466 mode=indexing
                        n296 = local read "xl"() -> (w482:dbl[])
                        n297 = local read "yl"() -> (w480:dbl[])
                        n298 = Subtract(x=w482, y=w481) -> (x-y=w478:dbl[])
                        n299 = Subtract(x=w479, y=w480) -> (x-y=w477:dbl[])
                        n300 = Square(x=w478) -> (x^2=w476:dbl[])
                        n301 = Square(x=w477) -> (x^2=w475:dbl[])
                        n302 = Add(x=w476, y=w475) -> (x+y=w474:dbl[])
                        n303 = Square Root(x=w474) -> (sqrt(x)=w473:dbl[])
                        n304 = Array Max & Min(array=w473) -> (min value=w472:dbl)  [unwired: 3 out]
                      }
                      n305 = Greater?(x=w466, y=1.0) -> (0:w458:bool[])
                      n306 = Boolean To (0,1)(Boolean=w458) -> (0, 1=w457:i16[])
                      n307 = local read "xr"() -> (w462:dbl[])
                      n308 = local read "yr"() -> (w461:dbl[])
                      n309 = To Long Integer(number=w457) -> (32bit integer=w456:i32[])
                      n310 = Build Cluster Array(w458, w462, w461) -> (w460:T6)
                      n311 = Add Array Elements(numeric array=w456) -> (sum=w455:i32)
                      n312 = Sort 1D Array(array=w460) -> (sorted array=w459:T6)
                      n313 = Reverse 1D Array(array=w459) -> (reversed array=w454:T6)
                      n314 = for {
                        N: w455 -> [_]
                        tunnel: w454 -> [w471] mode=indexing
                        tunnel: [w470] -> w465 mode=indexing
                        tunnel: [w469] -> w464 mode=indexing
                        n315 = Unbundle(w471) -> ("Rotational position"=w470:dbl, "Rotational position"=w469:dbl)  [unwired: 1 out]
                      }
                      n316 = local write "xr"(w465) -> ()
                      n317 = local write "yr"(w464) -> ()
                    }
                    frame True {
                    }
                  }
                }
                frame #1 {
                  n318 = local read "xr"() -> (w484:dbl[])
                  n319 = Empty Array?(array=w484) -> (empty?=w483:bool)
                  n320 = case shown="False" w483 {
                    frame False {
                      n321 = local read "xl"() -> (w500:dbl[])
                      n322 = local read "yl"() -> (w499:dbl[])
                      n323 = for {
                        tunnel: w500 -> [w513] mode=indexing
                        tunnel: w499 -> [w511] mode=indexing
                        tunnel: [w504] -> w486 mode=indexing
                        n324 = local read "xr"() -> (w514:dbl[])
                        n325 = local read "yr"() -> (w512:dbl[])
                        n326 = Subtract(x=w514, y=w513) -> (x-y=w510:dbl[])
                        n327 = Subtract(x=w511, y=w512) -> (x-y=w509:dbl[])
                        n328 = Square(x=w510) -> (x^2=w508:dbl[])
                        n329 = Square(x=w509) -> (x^2=w507:dbl[])
                        n330 = Add(x=w508, y=w507) -> (x+y=w506:dbl[])
                        n331 = Square Root(x=w506) -> (sqrt(x)=w505:dbl[])
                        n332 = Array Max & Min(array=w505) -> (min value=w504:dbl)  [unwired: 3 out]
                      }
                      n333 = Sort 1D Array(array=w486) -> (sorted array=→"sorted array":dbl[])
                      n334 = Greater?(x=w486, y=1.0) -> (0:w493:bool[])
                      n335 = Boolean To (0,1)(Boolean=w493) -> (0, 1=w492:i16[])
                      n336 = local read "xl"() -> (w497:dbl[])
                      n337 = local read "yl"() -> (w496:dbl[])
                      n338 = To Long Integer(number=w492) -> (32bit integer=w491:i32[])
                      n339 = Build Cluster Array(w493, w497, w496) -> (w495:T6)
                      n340 = Add Array Elements(numeric array=w491) -> (sum=w490:i32)
                      n341 = Sort 1D Array(array=w495) -> (sorted array=w494:T6)
                      n342 = Reverse 1D Array(array=w494) -> (reversed array=w489:T6)
                      n343 = for {
                        N: w490 -> [_]
                        tunnel: w489 -> [w503] mode=indexing
                        tunnel: [w502] -> w487 mode=indexing
                        tunnel: [w501] -> w488 mode=indexing
                        n344 = Unbundle(w503) -> ("Rotational position"=w502:dbl, "Rotational position"=w501:dbl)  [unwired: 1 out]
                      }
                      n345 = local write "xl"(w487) -> ()
                      n346 = local write "yl"(w488) -> ()
                    }
                    frame True {
                    }
                  }
                }
                frame #2 {
                  n347 = local read "yr"() -> (w516:dbl[])
                  n348 = local read "xl"() -> (w528:dbl[])
                  n349 = local read "yl"() -> (w527:dbl[])
                  n350 = local read "xr"() -> (w515:dbl[])
                  n351 = for {
                    tunnel: w528 -> [w562] mode=indexing
                    tunnel: w527 -> [w561] mode=indexing
                    tunnel: w528 -> [w567]
                    tunnel: w527 -> [w566]
                    shift-right: [w559] -> w525
                    shift-left: dbl[][] [] -> [w558]
                    n352 = Subtract(x=w567, y=w562) -> (x-y=w556:dbl[])
                    n353 = Subtract(x=w561, y=w566) -> (x-y=w576:dbl[])
                    n354 = Build Array(w562, w561) -> (w560:dbl[])
                    n355 = Multiply(x=2.0, y=w556) -> (x*y=w555:dbl[])
                    n356 = Square(x=w555) -> (x^2=w575:dbl[])
                    n357 = Square(x=w576) -> (x^2=w574:dbl[])
                    n358 = Add(x=w575, y=w574) -> (x+y=w573:dbl[])
                    n359 = Square Root(x=w573) -> (sqrt(x)=w572:dbl[])
                    n360 = Less?(x=w572, y=0.4) -> (x < y?=w570:bool[])
                    n361 = Boolean To (0,1)(Boolean=w570) -> (0, 1=w569:i16[])
                    n362 = To Long Integer(number=w569) -> (32bit integer=w568:i32[])
                    n363 = Add Array Elements(numeric array=w568) -> (sum=w565:i32)
                    n364 = Greater?(x=w565, y=3) -> (0:w563:bool)
                    n365 = case shown="True" w563 {
                      tunnel: w560 -> [_ w580]
                      tunnel: [w577 w579] -> w559
                      tunnel: w558 -> [w577 w578]
                      frame False {
                      }
                      frame True {
                        n366 = Build Array (concatenate)(w578, w580) -> (w579:dbl[][])
                      }
                    }
                  }
                  n367 = for {
                    tunnel: w515 -> [w536] mode=indexing
                    tunnel: w516 -> [w535] mode=indexing
                    tunnel: w515 -> [w541]
                    tunnel: w516 -> [w540]
                    shift-right: [w533] -> w518
                    shift-left: dbl[][] [] -> [w532]
                    n368 = Subtract(x=w541, y=w536) -> (x-y=w530:dbl[])
                    n369 = Subtract(x=w535, y=w540) -> (x-y=w550:dbl[])
                    n370 = Build Array(w536, w535) -> (w534:dbl[])
                    n371 = Multiply(x=2.0, y=w530) -> (x*y=w529:dbl[])
                    n372 = Square(x=w529) -> (x^2=w549:dbl[])
                    n373 = Square(x=w550) -> (x^2=w548:dbl[])
                    n374 = Add(x=w549, y=w548) -> (x+y=w547:dbl[])
                    n375 = Square Root(x=w547) -> (sqrt(x)=w546:dbl[])
                    n376 = Less?(x=w546, y=0.4) -> (x < y?=w544:bool[])
                    n377 = Boolean To (0,1)(Boolean=w544) -> (0, 1=w543:i16[])
                    n378 = To Long Integer(number=w543) -> (32bit integer=w542:i32[])
                    n379 = Add Array Elements(numeric array=w542) -> (sum=w539:i32)
                    n380 = Greater?(x=w539, y=3) -> (0:w537:bool)
                    n381 = case shown="False" w537 {
                      tunnel: w534 -> [_ w554]
                      tunnel: [w551 w553] -> w533
                      tunnel: w532 -> [w551 w552]
                      frame False {
                      }
                      frame True {
                        n382 = Build Array (concatenate)(w552, w554) -> (w553:dbl[][])
                      }
                    }
                  }
                  n383 = Index Array(array=w525, index (col) #1=0 ("disabled index (col)")) -> (element #1=w523:dbl[], element #2=w522:dbl[])  [unwired: 3 in]
                  n384 = Index Array(array=w518, index (col) #1=0 ("disabled index (col)")) -> (element #1=w520:dbl[], element #2=w521:dbl[])  [unwired: 3 in]
                  n385 = local write "xl"(w523) -> ()
                  n386 = local write "yl"(w522) -> ()
                  n387 = local write "xr"(w520) -> ()
                  n388 = local write "yr"(w521) -> ()
                }
              }
            }
            frame Disabled {
            }
          }
        }
        frame #6 {
          n389 = global read "G_ALL.vi" "mission num"() -> (w587:i32)
          n390 = case shown="2, 4, 6" w587 {
            tunnel: [_ TRUE] -> w586
            frame 0, Default {
            }
            frame 2, 4, 6 {
            }
          }
          n391 = local read "x"() -> (w594:dbl[])
          n392 = local read "xr"() -> (w593:dbl[])
          n393 = local read "x"() -> (w599:dbl[])
          n394 = local read "xl"() -> (w600:dbl[])
          n395 = Select(t=w599, s=w586, f=w600) -> (s? t:f=w598:dbl[])
          n396 = Select(t=w594, s=w586, f=w593) -> (s? t:f=w591:dbl[])
          n397 = local read "y"() -> (w589:dbl[])
          n398 = local read "yr"() -> (w590:dbl[])
          n399 = local read "y"() -> (w597:dbl[])
          n400 = local read "yl"() -> (w596:dbl[])
          n401 = Empty Array?(array=w591) -> (empty?=w592:bool)
          n402 = Empty Array?(array=w598) -> (empty?=w601:bool)
          n403 = Select(t=w597, s=w586, f=w596) -> (s? t:f=w595:dbl[])
          n404 = Select(t=w589, s=w586, f=w590) -> (s? t:f=w588:dbl[])
          n405 = case shown="False" w592 {
            tunnel: [w685 _] -> w626
            tunnel: [w684 _] -> w625
            tunnel: [w683 _] -> w624
            tunnel: [w682 _] -> w622
            tunnel: w591 -> [w658 _]
            tunnel: w588 -> [w657 _]
            frame False {
              n406 = local read "d_safe front"() -> (w660:dbl)
              n407 = local read "h_path"() -> (w659:dbl[])
              n408 = local read "d_safe"() -> (w644:dbl)
              n409 = local read "h_rf"() -> (w646:dbl[])
              n410 = local read "x_rf"() -> (w680:dbl[])
              n411 = local read "y_rf"() -> (w681:dbl[])
              n412 = local read "y_rr"() -> (w678:dbl[])
              n413 = local read "x_rr"() -> (w679:dbl[])
              n414 = for {
                tunnel: w658 -> [w722]
                tunnel: w657 -> [w721]
                tunnel: w681 -> [w735] mode=indexing
                tunnel: w680 -> [w719] mode=indexing
                tunnel: w659 -> [w711] mode=indexing
                tunnel: [w716] -> w648 mode=indexing
                tunnel: w660 -> [w699]
                tunnel: [w728] -> w650 mode=indexing
                tunnel: [w700] -> w636 mode=indexing
                tunnel: w679 -> [w724] mode=indexing
                tunnel: w678 -> [w723] mode=indexing
                tunnel: w646 -> [w702] mode=indexing
                tunnel: [w701] -> w645 mode=indexing
                tunnel: w644 -> [w698]
                n415 = Subtract(x=w722, y=w719) -> (x-y=w734:dbl[])
                n416 = Subtract(x=w721, y=w735) -> (x-y=w733:dbl[])
                n417 = Subtract(x=w722, y=w724) -> (x-y=w715:dbl[])
                n418 = Subtract(x=w721, y=w723) -> (x-y=w714:dbl[])
                n419 = call "headingoperater.vi"("h1"=w702, "h2"=1.5707963267948966) -> ("h2-h1"=w705:dbl)  [unwired: 8 in, 1 out]
                n420 = call "headingoperater.vi"("h1"=w711, "h2"=1.5707963267948966) -> ("h2-h1"=w710:dbl)  [unwired: 8 in, 1 out]
                n421 = Square(x=w734) -> (x^2=w731:dbl[])
                n422 = Square(x=w733) -> (x^2=w732:dbl[])
                n423 = Square(x=w714) -> (x^2=w713:dbl[])
                n424 = Square(x=w715) -> (x^2=w712:dbl[])
                n425 = Add(x=w731, y=w732) -> (x+y=w730:dbl[])
                n426 = Add(x=w713, y=w712) -> (x+y=w725:dbl[])
                n427 = call "headingoperater.vi"("h1"=1.5707963267948966, "h2"=w705) -> ("h2+h1"=w701:dbl)  [unwired: 8 in, 1 out]
                n428 = call "headingoperater.vi"("h1"=1.5707963267948966, "h2"=w710) -> ("h2+h1"=w716:dbl)  [unwired: 8 in, 1 out]
                n429 = Square Root(x=w730) -> (sqrt(x)=w729:dbl[])
                n430 = Square Root(x=w725) -> (sqrt(x)=w726:dbl[])
                n431 = Array Max & Min(array=w729) -> (min value=w718:dbl)  [unwired: 3 out]
                n432 = Array Max & Min(array=w726) -> (min value=w727:dbl)  [unwired: 3 out]
                n433 = Subtract(x=w699, y=w718) -> (x-y=w706:dbl)
                n434 = Subtract(x=w698, y=w727) -> (x-y=w707:dbl)
                n435 = Max & Min(x=w706, y=0.0) -> (max(x,y)=w728:dbl)  [unwired: 1 out]
                n436 = Max & Min(x=w707, y=0.0) -> (max(x,y)=w700:dbl)  [unwired: 1 out]
              }
              n437 = Add Array Elements(numeric array=w636) -> (sum=w662:dbl)
              n438 = Not Equal To 0?(x=w636) -> (x != 0?=w637:bool[])
              n439 = Polar To Re/Im(2:w648, 3:w636) -> (0:w674:dbl[], 1:w675:dbl[])
              n440 = disable-structure shown="Enabled" {
                disable-tunnel: w650 -> [w687 w697]
                disable-tunnel: w645 -> [w686 w694]
                disable-tunnel: [w687 w691] -> w649
                disable-tunnel: [w686 w689] -> w647
                frame Disabled {
                }
                frame Enabled {
                  n441 = local read "size limit"() -> (w693:i32)
                  n442 = local read "idxfront"() -> (w688:i32)
                  n443 = Array Subset(array=w697, index=0, length=w693) -> (w692:dbl[])
                  n444 = Array Subset(array=w694, index=0, length=w693) -> (w690:dbl[])
                  n445 = Array Subset(array=w692, index=w688) -> (w691:dbl[])  [unwired: 1 in]
                  n446 = Array Subset(array=w690, index=w688) -> (w689:dbl[])  [unwired: 1 in]
                }
              }
              n447 = Boolean To (0,1)(Boolean=w637) -> (0, 1=w638:i16[])
              n448 = Add Array Elements(numeric array=w675) -> (sum=w677:dbl)
              n449 = Add Array Elements(numeric array=w674) -> (sum=w676:dbl)
              n450 = To Long Integer(number=w638) -> (32bit integer=w639:i32[])
              n451 = Add Array Elements(numeric array=w639) -> (sum=w635:i32)
              n452 = local read "gap"() -> (w655:dbl)
              n453 = Max & Min(x=w635, y=1) -> (max(x,y)=w634:i32)  [unwired: 1 out]
              n454 = Divide(x=w662, y=w634) -> (x/y=w685:dbl)
              n455 = Divide(x=w677, y=w634) -> (x/y=w671:dbl)
              n456 = Divide(x=w676, y=w634) -> (x/y=w669:dbl)
              n457 = local read "af"() -> (w656:dbl)
              n458 = Divide(x=w655, y=w656) -> (x/y=w654:dbl)
              n459 = Multiply(x=w649, y=w654) -> (x*y=w643:dbl[])
              n460 = Add Array Elements(numeric array=w643) -> (sum=w661:dbl)
              n461 = Not Equal To 0?(x=w643) -> (x != 0?=w642:bool[])
              n462 = Polar To Re/Im(2:w647, 3:w643) -> (0:w651:dbl[], 1:w652:dbl[])
              n463 = Boolean To (0,1)(Boolean=w642) -> (0, 1=w641:i16[])
              n464 = Add Array Elements(numeric array=w652) -> (sum=w672:dbl)
              n465 = Add Array Elements(numeric array=w651) -> (sum=w673:dbl)
              n466 = To Long Integer(number=w641) -> (32bit integer=w640:i32[])
              n467 = Add Array Elements(numeric array=w640) -> (sum=w631:i32)
              n468 = Max & Min(x=w631, y=1) -> (max(x,y)=w630:i32)  [unwired: 1 out]
              n469 = Divide(x=w661, y=w630) -> (x/y=w684:dbl)
              n470 = Divide(x=w672, y=w630) -> (x/y=w670:dbl)
              n471 = Divide(x=w673, y=w630) -> (x/y=w653:dbl)
              n472 = Compound Arithmetic op=ADD(w671, w670) -> (w666:dbl)
              n473 = Compound Arithmetic op=ADD(w669, w653) -> (w663:dbl)
              n474 = Not A Number/Path/Refnum?(number/path/refnum=w666) -> (NaN/Path/Refnum?=w667:bool)
              n475 = Not A Number/Path/Refnum?(number/path/refnum=w663) -> (NaN/Path/Refnum?=w665:bool)
              n476 = Select(t=0.0, s=w667, f=w666) -> (s? t:f=w683:dbl)
              n477 = Select(t=0.0, s=w665, f=w663) -> (s? t:f=w682:dbl)
            }
            frame True {
            }
          }
          "rr_shift" <- w626
          "rf_shift" <- w625
          n478 = case shown="False" w601 {
            tunnel: [w791 _] -> w628
            tunnel: [w790 _] -> w627
            tunnel: [w789 _] -> w623
            tunnel: [w788 _] -> w621
            tunnel: w598 -> [w765 _]
            tunnel: w595 -> [w764 _]
            frame False {
              n479 = local read "h_path"() -> (w787:dbl[])
              n480 = local read "h_lf"() -> (w754:dbl[])
              n481 = local read "y_lf"() -> (w783:dbl[])
              n482 = local read "y_lr"() -> (w785:dbl[])
              n483 = local read "x_lf"() -> (w784:dbl[])
              n484 = local read "x_lr"() -> (w786:dbl[])
              n485 = for {
                tunnel: w765 -> [w829]
                tunnel: w764 -> [w828]
                tunnel: w787 -> [w816] mode=indexing
                tunnel: "d_safe front" -> [w830]
                tunnel: [w821] -> w753 mode=indexing
                tunnel: [w838] -> w757 mode=indexing
                tunnel: [w810] -> w739 mode=indexing
                tunnel: w786 -> [w827] mode=indexing
                tunnel: w785 -> [w826] mode=indexing
                tunnel: w784 -> [w825] mode=indexing
                tunnel: w783 -> [w824] mode=indexing
                tunnel: w754 -> [w806] mode=indexing
                tunnel: [w805] -> w752 mode=indexing
                tunnel: "d_safe" -> [w804]
                n486 = Subtract(x=w828, y=w824) -> (x-y=w832:dbl[])
                n487 = Subtract(x=w829, y=w825) -> (x-y=w831:dbl[])
                n488 = Subtract(x=w828, y=w826) -> (x-y=w819:dbl[])
                n489 = Subtract(x=w829, y=w827) -> (x-y=w820:dbl[])
                n490 = call "headingoperater.vi"("h1"=w806, "h2"=1.5707963267948966) -> ("h2-h1"=w809:dbl)  [unwired: 8 in, 1 out]
                n491 = call "headingoperater.vi"("h1"=w816, "h2"=1.5707963267948966) -> ("h2-h1"=w815:dbl)  [unwired: 8 in, 1 out]
                n492 = Square(x=w831) -> (x^2=w834:dbl[])
                n493 = Square(x=w832) -> (x^2=w833:dbl[])
                n494 = Square(x=w819) -> (x^2=w818:dbl[])
                n495 = Square(x=w820) -> (x^2=w817:dbl[])
                n496 = Add(x=w834, y=w833) -> (x+y=w835:dbl[])
                n497 = Add(x=w818, y=w817) -> (x+y=w841:dbl[])
                n498 = call "headingoperater.vi"("h1"=1.5707963267948966, "h2"=w809) -> ("h2-h1"=w805:dbl)  [unwired: 8 in, 1 out]
                n499 = call "headingoperater.vi"("h1"=1.5707963267948966, "h2"=w815) -> ("h2-h1"=w821:dbl)  [unwired: 8 in, 1 out]
                n500 = Square Root(x=w835) -> (sqrt(x)=w836:dbl[])
                n501 = Square Root(x=w841) -> (sqrt(x)=w840:dbl[])
                n502 = Array Max & Min(array=w836) -> (min value=w837:dbl)  [unwired: 3 out]
                n503 = Array Max & Min(array=w840) -> (min value=w839:dbl)  [unwired: 3 out]
                n504 = Subtract(x=w830, y=w837) -> (x-y=w811:dbl)
                n505 = Subtract(x=w804, y=w839) -> (x-y=w814:dbl)
                n506 = Max & Min(x=w811, y=0.0) -> (max(x,y)=w838:dbl)  [unwired: 1 out]
                n507 = Max & Min(x=w814, y=0.0) -> (max(x,y)=w810:dbl)  [unwired: 1 out]
              }
              n508 = Add Array Elements(numeric array=w739) -> (sum=w767:dbl)
              n509 = Not Equal To 0?(x=w739) -> (x != 0?=w743:bool[])
              n510 = Polar To Re/Im(2:w753, 3:w739) -> (0:w779:dbl[], 1:w780:dbl[])
              n511 = disable-structure shown="Enabled" {
                disable-tunnel: w757 -> [w792 w801]
                disable-tunnel: [w793 w795] -> w755
                disable-tunnel: w752 -> [w793 w800]
                disable-tunnel: [w792 w797] -> w756
                frame Disabled {
                }
                frame Enabled {
                  n512 = local read "size limit"() -> (w799:i32)
                  n513 = local read "idxfront"() -> (w794:i32)
                  n514 = Array Subset(array=w801, index=0, length=w799) -> (w798:dbl[])
                  n515 = Array Subset(array=w800, index=0, length=w799) -> (w796:dbl[])
                  n516 = Array Subset(array=w798, index=w794) -> (w797:dbl[])  [unwired: 1 in]
                  n517 = Array Subset(array=w796, index=w794) -> (w795:dbl[])  [unwired: 1 in]
                }
              }
              n518 = Boolean To (0,1)(Boolean=w743) -> (0, 1=w742:i16[])
              n519 = Add Array Elements(numeric array=w780) -> (sum=w782:dbl)
              n520 = Add Array Elements(numeric array=w779) -> (sum=w781:dbl)
              n521 = To Long Integer(number=w742) -> (32bit integer=w741:i32[])
              n522 = Add Array Elements(numeric array=w741) -> (sum=w740:i32)
              n523 = local read "gap"() -> (w763:dbl)
              n524 = Max & Min(x=w740, y=1) -> (max(x,y)=w738:i32)  [unwired: 1 out]
              n525 = Divide(x=w767, y=w738) -> (x/y=w791:dbl)
              n526 = Divide(x=w782, y=w738) -> (x/y=w776:dbl)
              n527 = Divide(x=w781, y=w738) -> (x/y=w774:dbl)
              n528 = local read "af"() -> (w762:dbl)
              n529 = Divide(x=w763, y=w762) -> (x/y=w760:dbl)
              n530 = Multiply(x=w756, y=w760) -> (x*y=w745:dbl[])
              n531 = Add Array Elements(numeric array=w745) -> (sum=w766:dbl)
              n532 = Not Equal To 0?(x=w745) -> (x != 0?=w749:bool[])
              n533 = Polar To Re/Im(2:w755, 3:w745) -> (0:w758:dbl[], 1:w759:dbl[])
              n534 = Boolean To (0,1)(Boolean=w749) -> (0, 1=w748:i16[])
              n535 = Add Array Elements(numeric array=w759) -> (sum=w777:dbl)
              n536 = Add Array Elements(numeric array=w758) -> (sum=w778:dbl)
              n537 = To Long Integer(number=w748) -> (32bit integer=w747:i32[])
              n538 = Add Array Elements(numeric array=w747) -> (sum=w746:i32)
              n539 = Max & Min(x=w746, y=1) -> (max(x,y)=w744:i32)  [unwired: 1 out]
              n540 = Divide(x=w766, y=w744) -> (x/y=w790:dbl)
              n541 = Divide(x=w777, y=w744) -> (x/y=w775:dbl)
              n542 = Divide(x=w778, y=w744) -> (x/y=w761:dbl)
              n543 = Compound Arithmetic op=ADD(w776, w775) -> (w771:dbl)
              n544 = Compound Arithmetic op=ADD(w774, w761) -> (w768:dbl)
              n545 = Not A Number/Path/Refnum?(number/path/refnum=w771) -> (NaN/Path/Refnum?=w772:bool)
              n546 = Not A Number/Path/Refnum?(number/path/refnum=w768) -> (NaN/Path/Refnum?=w770:bool)
              n547 = Select(t=0.0, s=w772, f=w771) -> (s? t:f=w789:dbl)
              n548 = Select(t=0.0, s=w770, f=w768) -> (s? t:f=w788:dbl)
            }
            frame True {
            }
          }
          "lr_shift" <- w628
          "lf_shift" <- w627
          n549 = Add(x=w624, y=w623) -> (x+y=w609:dbl)
          n550 = Add(x=w622, y=w621) -> (x+y=w603:dbl)
          n551 = Absolute Value(x=w609) -> (abs(x)=w613:dbl)
          n552 = Absolute Value(x=w603) -> (abs(x)=w604:dbl)
          n553 = Less?(x=w613, y=0.0001) -> (x < y?=w611:bool)
          n554 = Less?(x=w604, y=0.0001) -> (x < y?=w606:bool)
          n555 = Select(t=0.0, s=w611, f=w609) -> (s? t:f=w608:dbl)
          "x_shift" <- w608
          n556 = Select(t=0.0, s=w606, f=w603) -> (s? t:f=w602:dbl)
          "y_shift" <- w602
          n557 = Absolute Value(x="x limit") -> (abs(x)=w615:dbl)
          n558 = Absolute Value(x="y limit") -> (abs(x)=w581:dbl)
          n559 = Multiply(x=w608, y="x_gain") -> (x*y=w618:dbl)
          n560 = Negate(x=w615) -> (-x=w614:dbl)
          n561 = Negate(x=w581) -> (-x=w583:dbl)
          n562 = Multiply(x="y_gain", y=w602) -> (x*y=w585:dbl)
          n563 = In Range and Coerce(upper limit=w615, x=w618, lower limit=w614) -> (coerced(x)=w617:dbl)  [unwired: 1 out]
          n564 = In Range and Coerce(upper limit=w581, x=w585, lower limit=w583) -> (coerced(x)=w584:dbl)  [unwired: 1 out]
          n565 = global write "G_SEN.vi" "vision x shift"(w617) -> ()
          n566 = global write "G_SEN.vi" "vision y shift"(w584) -> ()
        }
        frame #7 {
          n567 = local read "R0"() -> (w891:dbl)
          n568 = local read "r"() -> (w890:dbl[])
          n569 = local read "rout"() -> (w881:dbl[])
          n570 = Reciprocal(x=w890) -> (1/x=w889:dbl[])
          n571 = Reciprocal(x=w891) -> (1/x=w888:dbl)
          n572 = Reciprocal(x=w881) -> (1/x=w882:dbl[])
          n573 = Threshold 1D Array(2:w888, 3:w889) -> (0:w880:dbl)  [unwired: 1 in]
          n574 = local read "rin"() -> (w887:dbl[])
          n575 = Interpolate 1D Array(1:w880, 2:w882) -> (0:w883:dbl)
          n576 = Reciprocal(x=w887) -> (1/x=w886:dbl[])
          n577 = Reciprocal(x=w883) -> (1/x=w879:dbl)
          n578 = Interpolate 1D Array(1:w880, 2:w886) -> (0:w885:dbl)
          n579 = local read "R0"() -> (w878:dbl)
          n580 = Absolute Value(x=w879) -> (abs(x)=w923:dbl)
          n581 = Reciprocal(x=w885) -> (1/x=w884:dbl)
          n582 = local read "size limit"() -> (w845:i32)
          n583 = Absolute Value(x=w878) -> (abs(x)=w933:dbl)
          n584 = local read "theta"() -> (w924:dbl[])
          n585 = Absolute Value(x=w884) -> (abs(x)=w928:dbl)
          n586 = local read "y_rf"() -> (w859:dbl[])
          n587 = local read "y_lf"() -> (w861:dbl[])
          n588 = local read "size limit"() -> (w851:i32)
          n589 = local read "idxfront"() -> (w842:i32)
          n590 = Array Subset(array=w861, index=0, length=w845) -> (w844:dbl[])
          n591 = Array Subset(array=w859, index=0, length=w845) -> (w843:dbl[])
          n592 = local read "theta"() -> (w934:dbl[])
          n593 = local read "theta"() -> (w927:dbl[])
          n594 = Polar To Re/Im(2:w924, 3:w923) -> (0:w920:dbl[], 1:w922:dbl[])
          n595 = local read "x_lf"() -> (w857:dbl[])
          n596 = local read "x_rf"() -> (w854:dbl[])
          n597 = local read "idxfront"() -> (w850:i32)
          n598 = local read "y_path"() -> (w903:dbl[])
          n599 = local read "y_shift"() -> (w868:dbl)
          n600 = local read "y_path"() -> (w869:dbl[])
          n601 = Array Subset(array=w857, index=0, length=w851) -> (w849:dbl[])
          n602 = Array Subset(array=w854, index=0, length=w851) -> (w848:dbl[])
          n603 = Add(x=w878, y=w922) -> (x+y=w921:dbl[])
          n604 = Array Subset(array=w844, index=w842) -> (w860:dbl[])  [unwired: 1 in]
          n605 = Array Subset(array=w843, index=w842) -> (w858:dbl[])  [unwired: 1 in]
          n606 = Polar To Re/Im(2:w934, 3:w933) -> (0:w930:dbl[], 1:w932:dbl[])
          n607 = Polar To Re/Im(2:w927, 3:w928) -> (0:w925:dbl[], 1:w929:dbl[])
          n608 = call "Convert to Dynamic Data12"("Array"=w920) -> ("Dynamic Data Type"=w914:dynamicdata)  [unwired: 3 in]
          n609 = local read "y_lr"() -> (w902:dbl[])
          n610 = local read "y_rr"() -> (w898:dbl[])
          n611 = local read "x_path"() -> (w913:dbl[])
          n612 = local read "x_shift"() -> (w872:dbl)
          n613 = local read "x_path"() -> (w873:dbl[])
          n614 = local read "y_car"() -> (w895:dbl[])
          n615 = Add(x=w878, y=w932) -> (x+y=w931:dbl[])
          n616 = Add(x=w878, y=w929) -> (x+y=w926:dbl[])
          n617 = Add(x=w868, y=w869) -> (x+y=w867:dbl[])
          n618 = Array Subset(array=w849, index=w850) -> (w856:dbl[])  [unwired: 1 in]
          n619 = Array Subset(array=w848, index=w850) -> (w855:dbl[])  [unwired: 1 in]
          n620 = call "Convert to Dynamic Data11"("Array"=w921) -> ("Dynamic Data Type"=w917:dynamicdata)  [unwired: 3 in]
          n621 = local read "x_lr"() -> (w905:dbl[])
          n622 = local read "x_rr"() -> (w901:dbl[])
          n623 = call "Convert to Dynamic Data8"("Array"=w930) -> ("Dynamic Data Type"=w916:dynamicdata)  [unwired: 3 in]
          n624 = call "Convert to Dynamic Data10"("Array"=w925) -> ("Dynamic Data Type"=w915:dynamicdata)  [unwired: 3 in]
          n625 = call "Convert to Dynamic Data15"("Array"=w903) -> ("Dynamic Data Type"=w908:dynamicdata)  [unwired: 3 in]
          n626 = call "Convert to Dynamic Data16"("Array"=w860) -> ("Dynamic Data Type"=w909:dynamicdata)  [unwired: 3 in]
          n627 = call "Convert to Dynamic Data17"("Array"=w902) -> ("Dynamic Data Type"=w906:dynamicdata)  [unwired: 3 in]
          n628 = call "Convert to Dynamic Data21"("Array"=w858) -> ("Dynamic Data Type"=w897:dynamicdata)  [unwired: 3 in]
          n629 = call "Convert to Dynamic Data22"("Array"=w898) -> ("Dynamic Data Type"=w896:dynamicdata)  [unwired: 3 in]
          n630 = local read "x_car"() -> (w893:dbl[])
          n631 = Merge Signals(w908, w909, w906, w897, w896) -> (w907:dynamicdata)
          n632 = Merge Signals(w916, w915, w914) -> (w874:dynamicdata)
          n633 = Add(x=w872, y=w873) -> (x+y=w871:dbl[])
          n634 = call "Convert to Dynamic Data7"("Array"=w931) -> ("Dynamic Data Type"=w919:dynamicdata)  [unwired: 3 in]
          n635 = call "Convert to Dynamic Data9"("Array"=w926) -> ("Dynamic Data Type"=w918:dynamicdata)  [unwired: 3 in]
          n636 = call "Convert to Dynamic Data13"("Array"=w913) -> ("Dynamic Data Type"=w912:dynamicdata)  [unwired: 3 in]
          n637 = call "Convert to Dynamic Data14"("Array"=w856) -> ("Dynamic Data Type"=w911:dynamicdata)  [unwired: 3 in]
          n638 = call "Convert to Dynamic Data18"("Array"=w905) -> ("Dynamic Data Type"=w904:dynamicdata)  [unwired: 3 in]
          n639 = call "Convert to Dynamic Data19"("Array"=w855) -> ("Dynamic Data Type"=w900:dynamicdata)  [unwired: 3 in]
          n640 = call "Convert to Dynamic Data20"("Array"=w901) -> ("Dynamic Data Type"=w899:dynamicdata)  [unwired: 3 in]
          n641 = call "Convert to Dynamic Data23"("Array"=w895) -> ("Dynamic Data Type"=w894:dynamicdata)  [unwired: 3 in]
          n642 = call "Convert to Dynamic Data26"("Array"=w867) -> ("Dynamic Data Type"=w866:dynamicdata)  [unwired: 3 in]
          n643 = local read "yl"() -> (w864:dbl[])
          n644 = local read "yr"() -> (w862:dbl[])
          n645 = local read "y"() -> (w877:dbl[])
          n646 = Merge Signals(w912, w911, w904, w900, w899) -> (w910:dynamicdata)
          n647 = Merge Signals(w919, w918, w917) -> (w875:dynamicdata)
          n648 = call "Convert to Dynamic Data24"("Array"=w893) -> ("Dynamic Data Type"=w892:dynamicdata)  [unwired: 3 in]
          n649 = call "Convert to Dynamic Data25"("Array"=w871) -> ("Dynamic Data Type"=w870:dynamicdata)  [unwired: 3 in]
          n650 = call "Convert to Dynamic Data4"("Array"=w864) -> ("Dynamic Data Type"=w937:dynamicdata)  [unwired: 3 in]
          n651 = call "Convert to Dynamic Data2"("Array"=w877) -> ("Dynamic Data Type"=w943:dynamicdata)  [unwired: 3 in]
          n652 = call "Convert to Dynamic Data6"("Array"=w862) -> ("Dynamic Data Type"=w935:dynamicdata)  [unwired: 3 in]
          n653 = local read "xl"() -> (w865:dbl[])
          n654 = local read "xr"() -> (w863:dbl[])
          n655 = local read "x"() -> (w876:dbl[])
          n656 = Merge Signals(w943, w937, w935, w874, w907, w894, w866) -> (w938:dynamicdata)
          n657 = call "Convert to Dynamic Data3"("Array"=w865) -> ("Dynamic Data Type"=w939:dynamicdata)  [unwired: 3 in]
          n658 = call "Convert to Dynamic Data"("Array"=w876) -> ("Dynamic Data Type"=w942:dynamicdata)  [unwired: 3 in]
          n659 = call "Convert to Dynamic Data5"("Array"=w863) -> ("Dynamic Data Type"=w936:dynamicdata)  [unwired: 3 in]
          n660 = Merge Signals(w942, w939, w936, w875, w910, w892, w870) -> (w940:dynamicdata)
          n661 = call "Build XY Graph"("Y Input"=w938, "X Input"=w940) -> ("XY Graph"=→"XY Graph":cluster{"X":dbl[], "Y":dbl[]}[])  [unwired: 8 in, 1 out]
        }
      }
    }
  }
